vi "ACQ_Data_viewer (Module).vi"(0 "ACQ full DATA file path":path caption="File path", 5 "ChipID list":u32[](array[numeric]) format="%.0x", 7 "quants events per chip":u32[](array[numeric]), 9 "ID summary":string, 11 "ACQ events fets":u32=80 caption="Acquired events") -> ()   [LabVIEW 2015, in "VIPM2.lvlib"]
doc: "<b>Acquisition Data viewer</b>\nInclou ACQ choose Chip Data_viewer.vi"
uses:
  VIPM2.lvlib
  <vilib>/Analysis/NI_AALBase.lvlib
panel:
  out "Valid data":bool
  out "Barra Load events":i32(slide)
  in  "X scale max.":dbl=150.0 min=0.0 max=1e+29 step=10.0
  in  "X scale min.":dbl=80.0 min=0.0 max=1e+29 step=10.0
  in  "Y scale":dbl=100.0 min=5.0 max=1e+29 step=10.0
  in  "Take image button":bool
  in  "Choose Chip button":bool
  in  "Close button":bool
  out "Total number of events":u32
  out "data time":string
  out "Chip ID":string
  out "Trigger histogram 99":T1(graph)
  out "Trigger histogram 98":T1(graph)
  out "Trigger histogram 97":T1(graph)
  out "Trigger histogram 96":T1(graph)
  out "Trigger histogram 95":T1(graph)
  out "Trigger histogram 94":T1(graph)
  out "Trigger histogram 93":T1(graph)
  out "Trigger histogram 92":T1(graph)
  out "Trigger histogram 91":T1(graph)
  out "Trigger histogram 90":T1(graph)
  out "Trigger histogram 89":T1(graph)
  out "Trigger histogram 88":T1(graph)
  out "Trigger histogram 87":T1(graph)
  out "Trigger histogram 86":T1(graph)
  out "Trigger histogram 85":T1(graph)
  out "Trigger histogram 84":T1(graph)
  out "Trigger histogram 83":T1(graph)
  out "Trigger histogram 82":T1(graph)
  out "Trigger histogram 81":T1(graph)
  out "Trigger histogram 80":T1(graph)
  out "Trigger histogram 79":T1(graph)
  out "Trigger histogram 78":T1(graph)
  out "Trigger histogram 77":T1(graph)
  out "Trigger histogram 76":T1(graph)
  out "Trigger histogram 75":T1(graph)
  out "Trigger histogram 74":T1(graph)
  out "Trigger histogram 73":T1(graph)
  out "Trigger histogram 72":T1(graph)
  out "Trigger histogram 71":T1(graph)
  out "Trigger histogram 70":T1(graph)
  out "Trigger histogram 69":T1(graph)
  out "Trigger histogram 68":T1(graph)
  out "Trigger histogram 67":T1(graph)
  out "Trigger histogram 66":T1(graph)
  out "Trigger histogram 65":T1(graph)
  out "Trigger histogram 64":T1(graph)
  out "Trigger histogram 63":T1(graph)
  out "Trigger histogram 62":T1(graph)
  out "Trigger histogram 61":T1(graph)
  out "Trigger histogram 60":T1(graph)
  out "Trigger histogram 59":T1(graph)
  out "Trigger histogram 58":T1(graph)
  out "Trigger histogram 57":T1(graph)
  out "Trigger histogram 56":T1(graph)
  out "Trigger histogram 55":T1(graph)
  out "Trigger histogram 54":T1(graph)
  out "Trigger histogram 53":T1(graph)
  out "Trigger histogram 52":T1(graph)
  out "Trigger histogram 51":T1(graph)
  out "Trigger histogram 50":T1(graph)
  out "Trigger histogram 49":T1(graph)
  out "Trigger histogram 48":T1(graph)
  out "Trigger histogram 47":T1(graph)
  out "Trigger histogram 46":T1(graph)
  out "Trigger histogram 45":T1(graph)
  out "Trigger histogram 44":T1(graph)
  out "Trigger histogram 43":T1(graph)
  out "Trigger histogram 42":T1(graph)
  out "Trigger histogram 41":T1(graph)
  out "Trigger histogram 40":T1(graph)
  out "Trigger histogram 39":T1(graph)
  out "Trigger histogram 38":T1(graph)
  out "Trigger histogram 37":T1(graph)
  out "Trigger histogram 36":T1(graph)
  out "Trigger histogram 35":T1(graph)
  out "Trigger histogram 34":T1(graph)
  out "Trigger histogram 33":T1(graph)
  out "Trigger histogram 32":T1(graph)
  out "Trigger histogram 31":T1(graph)
  out "Trigger histogram 30":T1(graph)
  out "Trigger histogram 29":T1(graph)
  out "Trigger histogram 28":T1(graph)
  out "Trigger histogram 27":T1(graph)
  out "Trigger histogram 26":T1(graph)
  out "Trigger histogram 25":T1(graph)
  out "Trigger histogram 24":T1(graph)
  out "Trigger histogram 23":T1(graph)
  out "Trigger histogram 22":T1(graph)
  out "Trigger histogram 21":T1(graph)
  out "Trigger histogram 20":T1(graph)
  out "Trigger histogram 19":T1(graph)
  out "Trigger histogram 18":T1(graph)
  out "Trigger histogram 17":T1(graph)
  out "Trigger histogram 16":T1(graph)
  out "Trigger histogram 15":T1(graph)
  out "Trigger histogram 14":T1(graph)
  out "Trigger histogram 13":T1(graph)
  out "Trigger histogram 12":T1(graph)
  out "Trigger histogram 11":T1(graph)
  out "Trigger histogram 10":T1(graph)
  out "Trigger histogram 09":T1(graph)
  out "Trigger histogram 08":T1(graph)
  out "Trigger histogram 07":T1(graph)
  out "Trigger histogram 06":T1(graph)
  out "Trigger histogram 05":T1(graph)
  out "Trigger histogram 04":T1(graph)
  out "Trigger histogram 03":T1(graph)
  out "Trigger histogram 01":T1(graph)
  out "Trigger histogram 00":T1(graph)
  out "Trigger histogram 02":T1(graph)
  out "100px Trigger Data":cluster{"1px Trigger Data":u16[]}[](array[cluster])
  # "99"
  # "98"
  # "97"
  # "96"
  # "95"
  # "94"
  # "93"
  # "92"
  # "91"
  # "90"
  # "89"
  # "88"
  # "87"
  # "86"
  # "85"
  # "84"
  # "83"
  # "82"
  # "81"
  # "80"
  # "79"
  # "78"
  # "77"
  # "76"
  # "75"
  # "74"
  # "73"
  # "72"
  # "71"
  # "70"
  # "69"
  # "68"
  # "67"
  # "66"
  # "65"
  # "64"
  # "63"
  # "62"
  # "61"
  # "60"
  # "59"
  # "58"
  # "57"
  # "56"
  # "55"
  # "54"
  # "53"
  # "52"
  # "51"
  # "50"
  # "49"
  # "48"
  # "47"
  # "46"
  # "45"
  # "44"
  # "43"
  # "42"
  # "41"
  # "40"
  # "39"
  # "38"
  # "37"
  # "36"
  # "35"
  # "34"
  # "33"
  # "32"
  # "31"
  # "30"
  # "29"
  # "28"
  # "27"
  # "26"
  # "25"
  # "24"
  # "23"
  # "22"
  # "21"
  # "20"
  # "19"
  # "18"
  # "17"
  # "16"
  # "15"
  # "14"
  # "13"
  # "12"
  # "11"
  # "10"
  # "09"
  # "08"
  # "07"
  # "06"
  # "05"
  # "04"
  # "03"
  # "01"
  # "00"
  # "02"
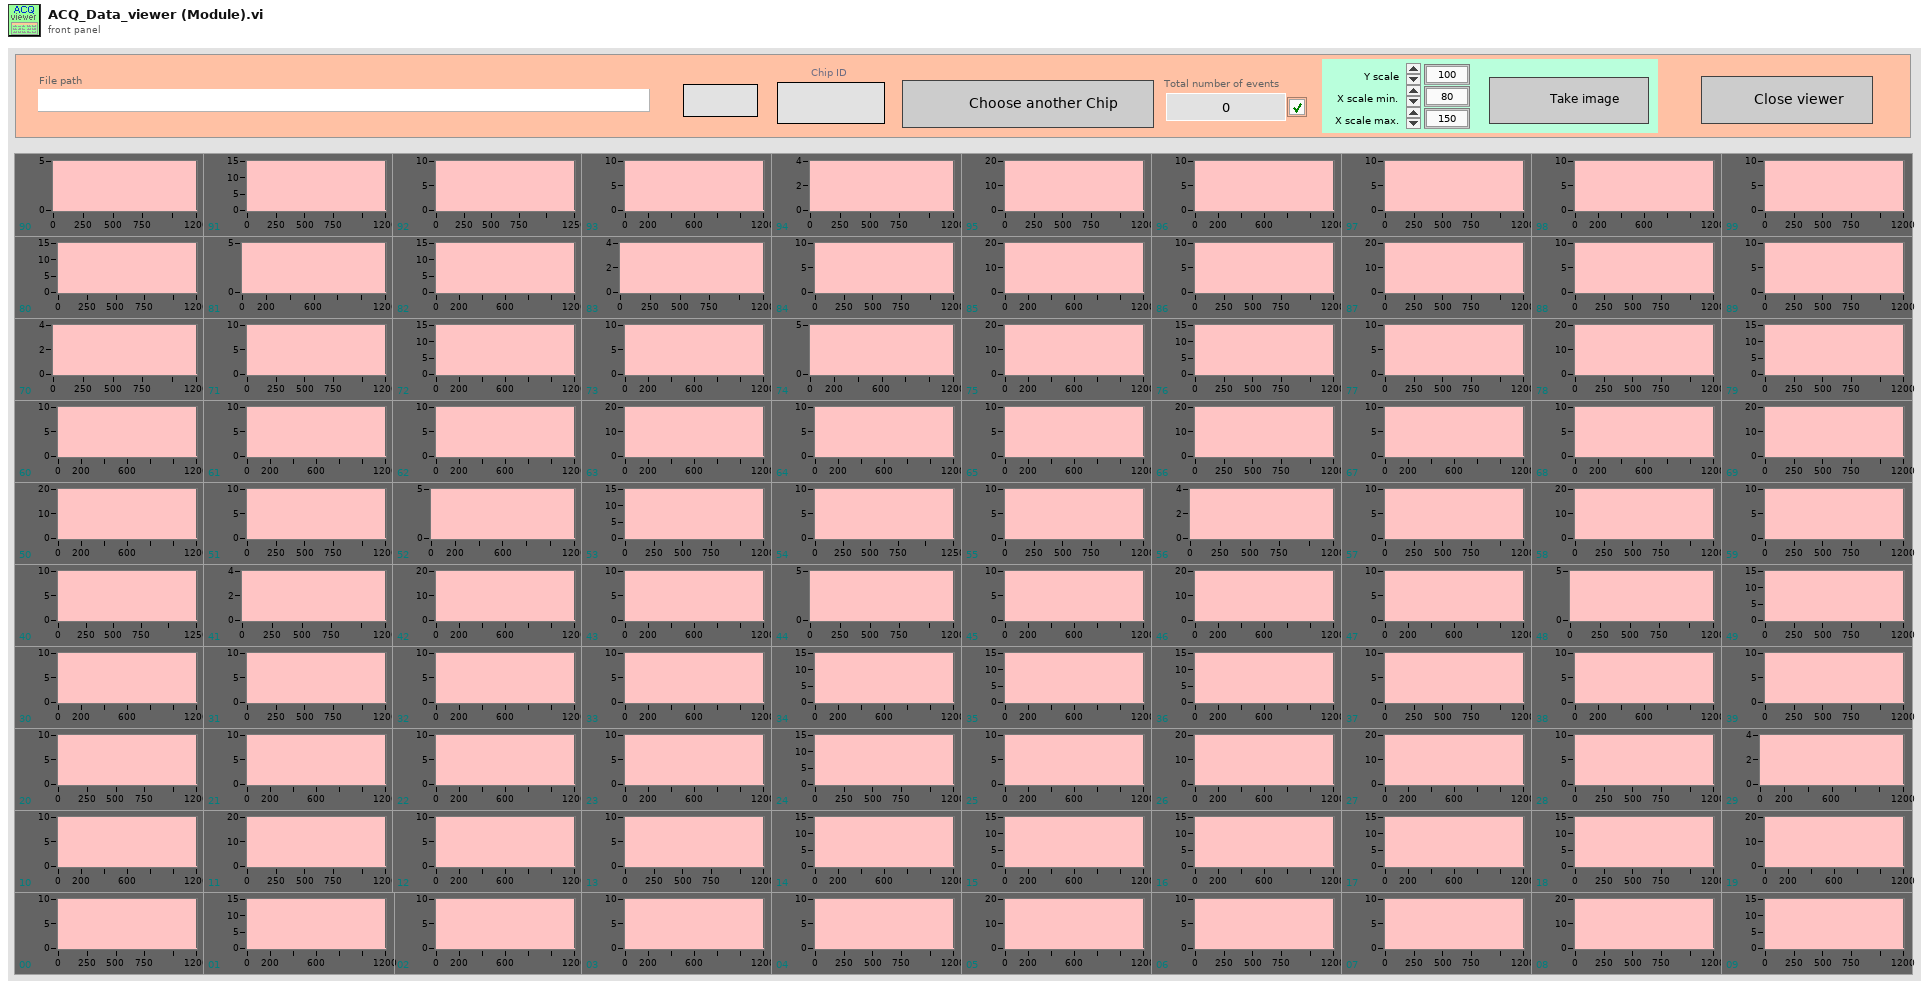
[diagram p1: front panel]
types:
  T1 = cluster{"X Values":dbl[], "Histogram: h(x)":i32[]}
  T2 = enum16{"big-endian, network order", "native, host order", "little-endian"}
  T3 = typedef "imagedata.ctl" = cluster{"image type":i32, "image depth":i32, "image":u8[], "mask":u8[], "colors":u32[], "Rectangle":cluster{"left":i16, "top":i16, "right":i16, "bottom":i16}}
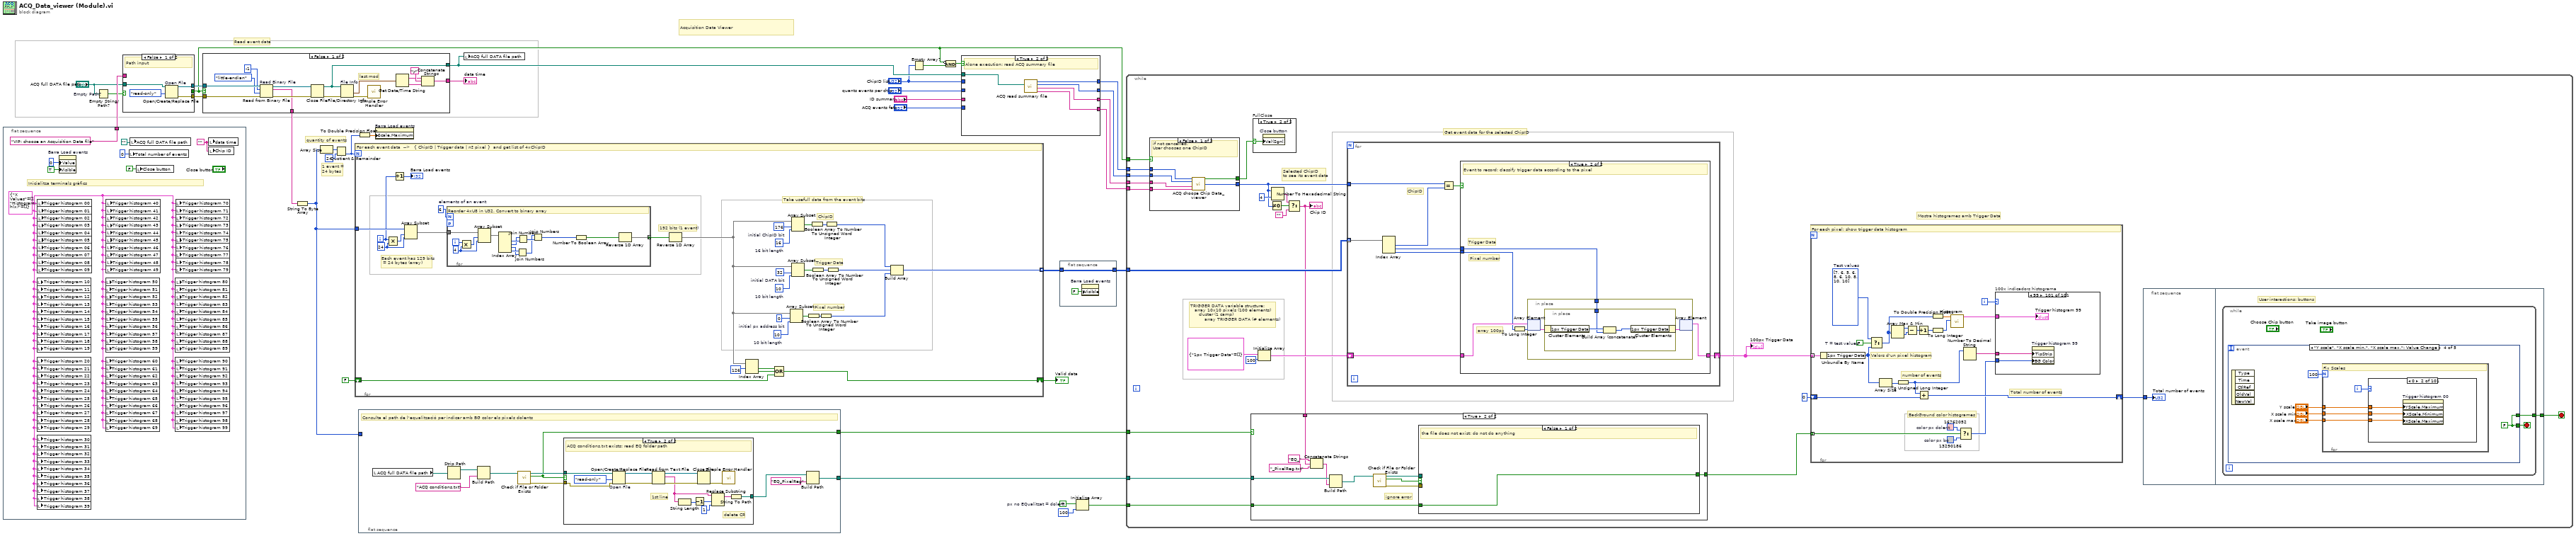
[diagram p0: block diagram]
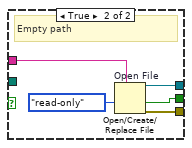
[diagram p3: hidden frame]
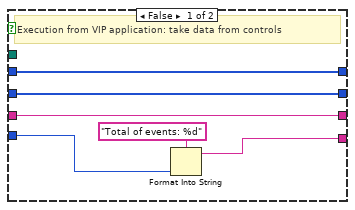
[diagram p5: hidden frame]
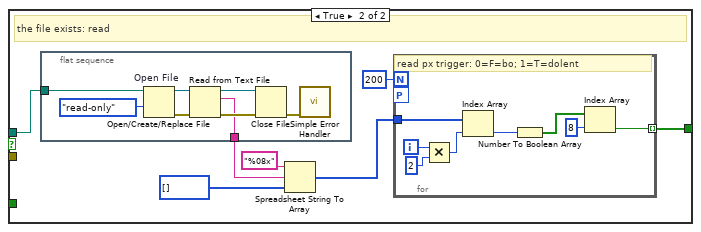
[diagram p8: hidden frame]
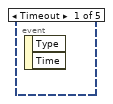
[diagram p10: hidden frame]
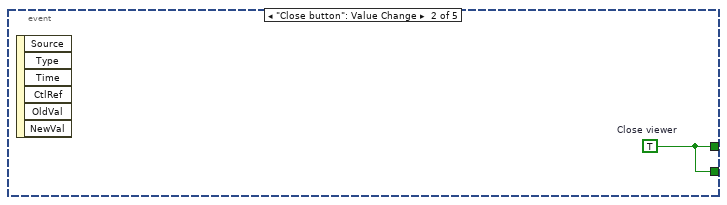
[diagram p11: hidden frame]
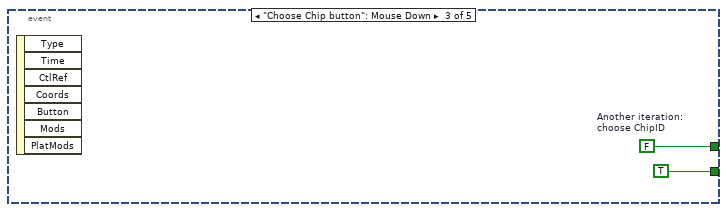
[diagram p12: hidden frame]
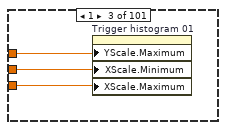
[diagram p14: hidden frame]
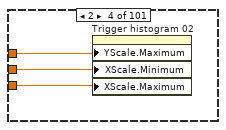
[diagram p15: hidden frame]
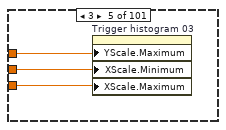
[diagram p16: hidden frame]
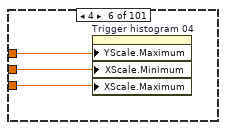
[diagram p17: hidden frame]
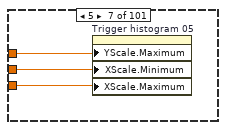
[diagram p18: hidden frame]
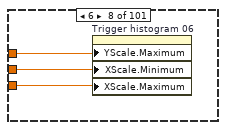
[diagram p19: hidden frame]
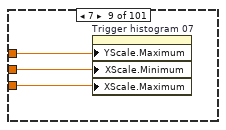
[diagram p20: hidden frame]
diagram:
  w4 = TRUE  # px no EQualitzat = dolent
  # "1 event =\n24 bytes"
  # "quantity of events"
  # "Read event data"
  # "Acquisition Data Viewer"
  n1 = flat-sequence {
    tunnel: ["VIP: choose an Acquisition Data file" ("prompt")] -> w30
    frame #0 {
      w37 = T1 {"X Values"=[], "Histogram: h(x)"=[]} ("Trigger histogram 00")
      w39 = ""
      # "Inicialitza terminals gràfics"
      n2 = local write "Trigger histogram 10"(w37) -> ()
      n3 = local write "Trigger histogram 11"(w37) -> ()
      n4 = local write "Trigger histogram 12"(w37) -> ()
      n5 = local write "Trigger histogram 13"(w37) -> ()
      n6 = local write "Trigger histogram 14"(w37) -> ()
      n7 = local write "Trigger histogram 15"(w37) -> ()
      n8 = local write "Trigger histogram 16"(w37) -> ()
      n9 = local write "Trigger histogram 17"(w37) -> ()
      n10 = local write "Trigger histogram 18"(w37) -> ()
      n11 = local write "Trigger histogram 19"(w37) -> ()
      n12 = local write "Trigger histogram 20"(w37) -> ()
      n13 = local write "Trigger histogram 21"(w37) -> ()
      n14 = local write "Trigger histogram 22"(w37) -> ()
      n15 = local write "Trigger histogram 23"(w37) -> ()
      n16 = local write "Trigger histogram 24"(w37) -> ()
      n17 = local write "Trigger histogram 25"(w37) -> ()
      n18 = local write "Trigger histogram 26"(w37) -> ()
      n19 = local write "Trigger histogram 27"(w37) -> ()
      n20 = local write "Trigger histogram 28"(w37) -> ()
      n21 = local write "Trigger histogram 29"(w37) -> ()
      n22 = local write "Trigger histogram 30"(w37) -> ()
      n23 = local write "Trigger histogram 31"(w37) -> ()
      n24 = local write "Trigger histogram 32"(w37) -> ()
      n25 = local write "Trigger histogram 33"(w37) -> ()
      n26 = local write "Trigger histogram 34"(w37) -> ()
      n27 = local write "Trigger histogram 35"(w37) -> ()
      n28 = local write "Trigger histogram 36"(w37) -> ()
      n29 = local write "Trigger histogram 37"(w37) -> ()
      n30 = local write "Trigger histogram 38"(w37) -> ()
      n31 = local write "Trigger histogram 39"(w37) -> ()
      n32 = local write "Trigger histogram 00"(w37) -> ()
      n33 = local write "Trigger histogram 01"(w37) -> ()
      n34 = local write "Trigger histogram 02"(w37) -> ()
      n35 = local write "Trigger histogram 03"(w37) -> ()
      n36 = local write "Trigger histogram 04"(w37) -> ()
      n37 = local write "Trigger histogram 05"(w37) -> ()
      n38 = local write "Trigger histogram 06"(w37) -> ()
      n39 = local write "Trigger histogram 07"(w37) -> ()
      n40 = local write "Trigger histogram 08"(w37) -> ()
      n41 = local write "Trigger histogram 09"(w37) -> ()
      n42 = property on="Barra Load events" class="Slide (strict)"("Value"=0 ("Barra Load events"), "Visible"=TRUE) -> ()  [unwired: 2 in, 2 out]
      n43 = local write "Trigger histogram 50"(w37) -> ()
      n44 = local write "Trigger histogram 51"(w37) -> ()
      n45 = local write "Trigger histogram 52"(w37) -> ()
      n46 = local write "Trigger histogram 53"(w37) -> ()
      n47 = local write "Trigger histogram 54"(w37) -> ()
      n48 = local write "Trigger histogram 55"(w37) -> ()
      n49 = local write "Trigger histogram 56"(w37) -> ()
      n50 = local write "Trigger histogram 57"(w37) -> ()
      n51 = local write "Trigger histogram 58"(w37) -> ()
      n52 = local write "Trigger histogram 59"(w37) -> ()
      n53 = local write "Trigger histogram 60"(w37) -> ()
      n54 = local write "Trigger histogram 61"(w37) -> ()
      n55 = local write "Trigger histogram 62"(w37) -> ()
      n56 = local write "Trigger histogram 63"(w37) -> ()
      n57 = local write "Trigger histogram 64"(w37) -> ()
      n58 = local write "Trigger histogram 65"(w37) -> ()
      n59 = local write "Trigger histogram 66"(w37) -> ()
      n60 = local write "Trigger histogram 67"(w37) -> ()
      n61 = local write "Trigger histogram 68"(w37) -> ()
      n62 = local write "Trigger histogram 69"(w37) -> ()
      n63 = local write "Trigger histogram 40"(w37) -> ()
      n64 = local write "Trigger histogram 41"(w37) -> ()
      n65 = local write "Trigger histogram 42"(w37) -> ()
      n66 = local write "Trigger histogram 43"(w37) -> ()
      n67 = local write "Trigger histogram 44"(w37) -> ()
      n68 = local write "Trigger histogram 45"(w37) -> ()
      n69 = local write "Trigger histogram 46"(w37) -> ()
      n70 = local write "Trigger histogram 47"(w37) -> ()
      n71 = local write "Trigger histogram 48"(w37) -> ()
      n72 = local write "Trigger histogram 49"(w37) -> ()
      n73 = local write "Total number of events"(u32 0 ("Total number of events")) -> ()
      n74 = local write "ACQ full DATA file path"(path "") -> ()
      n75 = local write "Close button"(FALSE ("Close button")) -> ()
      n76 = local write "Trigger histogram 80"(w37) -> ()
      n77 = local write "Trigger histogram 81"(w37) -> ()
      n78 = local write "Trigger histogram 82"(w37) -> ()
      n79 = local write "Trigger histogram 83"(w37) -> ()
      n80 = local write "Trigger histogram 84"(w37) -> ()
      n81 = local write "Trigger histogram 85"(w37) -> ()
      n82 = local write "Trigger histogram 86"(w37) -> ()
      n83 = local write "Trigger histogram 87"(w37) -> ()
      n84 = local write "Trigger histogram 88"(w37) -> ()
      n85 = local write "Trigger histogram 89"(w37) -> ()
      n86 = local write "Trigger histogram 90"(w37) -> ()
      n87 = local write "Trigger histogram 91"(w37) -> ()
      n88 = local write "Trigger histogram 92"(w37) -> ()
      n89 = local write "Trigger histogram 93"(w37) -> ()
      n90 = local write "Trigger histogram 94"(w37) -> ()
      n91 = local write "Trigger histogram 95"(w37) -> ()
      n92 = local write "Trigger histogram 96"(w37) -> ()
      n93 = local write "Trigger histogram 97"(w37) -> ()
      n94 = local write "Trigger histogram 98"(w37) -> ()
      n95 = local write "Trigger histogram 99"(w37) -> ()
      n96 = local write "Trigger histogram 70"(w37) -> ()
      n97 = local write "Trigger histogram 71"(w37) -> ()
      n98 = local write "Trigger histogram 72"(w37) -> ()
      n99 = local write "Trigger histogram 73"(w37) -> ()
      n100 = local write "Trigger histogram 74"(w37) -> ()
      n101 = local write "Trigger histogram 75"(w37) -> ()
      n102 = local write "Trigger histogram 76"(w37) -> ()
      n103 = local write "Trigger histogram 77"(w37) -> ()
      n104 = local write "Trigger histogram 78"(w37) -> ()
      n105 = local write "Trigger histogram 79"(w37) -> ()
      n106 = local write "data time"(w39) -> ()
      n107 = local write "Chip ID"(w39) -> ()
    }
  }
  n108 = Empty String/Path? "Empty Path?"(string/path="ACQ full DATA file path") -> (empty?=w29:bool)
  n109 = case shown="False" w29 {
    tunnel: [w44 w49] -> w33
    tunnel: [w43 w48] -> w32
    tunnel: [_ w47] -> w9
    tunnel: w30 -> [_ w46]
    tunnel: "ACQ full DATA file path" -> [w42 _]
    frame False {
      # "Path input"
      n110 = Open/Create/Replace File "Open File"(file path (use dialog)=w42, access (0:read/write)=enum16{"read/write", "read-only", "write-only"}."read-only") -> (refnum out=w43:refnum<file>, error out=w44:errorcluster)  [unwired: 4 in, 1 out]
    }
    frame True {
      # "Empty path"
      n111 = Open/Create/Replace File "Open File"(prompt=w46, access (0:read/write)=enum16{"read/write", "read-only", "write-only"}."read-only") -> (refnum out=w48:refnum<file>, cancelled=w47:bool, error out=w49:errorcluster)  [unwired: 4 in]
    }
  }
  n112 = case shown="False" w9 {
    tunnel: w33 -> [w65 _]
    tunnel: w32 -> [w64 _]
    tunnel: [w59 _] -> w25
    tunnel: [w52 _] -> w31
    tunnel: [w51 _] -> w20
    frame False {
      # "last mod"
      n113 = Read from Binary File "Read Binary File"(8:w65, 9:T2."little-endian" ("byte order (0:big-endian, network order)"), 10:-1 ("count (1)"), 11:w64) -> (0:w62:errorcluster, 2:w59:string, 3:w61:refnum<file>)  [unwired: 2 in, 1 out]
      n114 = Close File(refnum=w61, error in=w62) -> (path=w51:path, error out=w58:errorcluster)
      n115 = File/Directory Info "File Info"(path=w51, error in=w58) -> (last mod=w53:timestamp, error out=w57:errorcluster)  [unwired: 5 out]
      n116 = call <vilib>:"Simple Error Handler.vi"("error in (no error)"=w57) -> ()  [unwired: 4 in, 5 out]
      n117 = Get Date/Time String(seconds (now)=w53) -> (date string=w54:string, time string=w56:string)  [unwired: 2 in]
      n118 = Concatenate Strings(w54, "\r", w56) -> (w52:string)
    }
    frame True {
      # "Openning cancelled"
    }
  }
  "data time" <- w31
  n119 = String To Byte Array(string=w25) -> (unsigned byte array=w8:u8[])
  n120 = Array Size(array=w8) -> (size(s)=w26:i32)
  n121 = Quotient & Remainder(x=w26, y=24) -> (floor(x/y)=w23:i32)  [unwired: 1 out]
  n122 = for {
    N: w23 -> [_]
    tunnel: w8 -> [w91]
    tunnel: [w74] -> w21 mode=indexing
    shift-right: [w66] -> w1
    shift-left: FALSE -> [w67]
    i -> [w72]
    w80 = 10  # 10 bit length
    w81 = 0  # initial px address bit
    w85 = 10  # 10 bit length
    w84 = 32  # initial DATA bit
    w88 = 16  # 16 bit length
    w89 = 176  # initial ChipID bit
    w94 = 24 ("y")
    w95 = 6  # elements of an event
    # "Take usefull data from the event bits"
    # "Pixel number"
    # "Trigger Data"
    # "ChipID"
    # "192 bits (1 event)"
    # "Each event has 129 bits\n = 24 bytes (array)"
    # "For each event data  -->   { ChipID | Trigger data | nº pixel }  and get list of 4xChipID"
    n123 = Multiply(x=w72, y=w94) -> (x*y=w93:i32)
    n124 = Increment(x=w72) -> (x+1=→"Barra Load events":i32)
    n125 = Array Subset "Array Subset"(array=w91, index=w93, length=w94) -> (w92:u8[])
    n126 = for {
      N: w95 -> [_]
      tunnel: w92 -> [w108]
      workers-P: _ -> [_]
      tunnel: [w96] -> w90 mode=concatenating
      i -> [w109]
      w106 = 4 ("y")
      # "Reorder 4xU8 in U32. Convert to binary array"
      n127 = Multiply(x=w109, y=w106) -> (x*y=w107:i32)
      n128 = Array Subset "Array Subset"(array=w108, index=w107, length=w106) -> (w105:u8[])
      n129 = Index Array(array=w105) -> (element #1=w104:u8, element #2=w103:u8, element #3=w101:u8, element #4=w102:u8)  [unwired: 4 in]
      n130 = Join Numbers(hi=w102, lo=w101) -> ((hi.lo)=w99:u16)
      n131 = Join Numbers(hi=w103, lo=w104) -> ((hi.lo)=w100:u16)
      n132 = Join Numbers(hi=w99, lo=w100) -> ((hi.lo)=w97:u32)
      n133 = Number To Boolean Array(number=w97) -> (Boolean array=w98:bool[])
      n134 = Reverse 1D Array(array=w98) -> (reversed array=w96:bool[])
    }
    n135 = Reverse 1D Array(array=w90) -> (reversed array=w71:bool[])
    n136 = Index Array(array=w71, index #1=126 ("index")) -> (element #1=w69:bool, element #2=w68:bool)  [unwired: 1 in]
    n137 = Compound Arithmetic op=OR(w69, w68, w67) -> (w66:bool)
    n138 = Array Subset "Array Subset"(array=w71, index=w81, length=w80) -> (w79:bool[])
    n139 = Array Subset "Array Subset"(array=w71, index=w89, length=w88) -> (w87:bool[])
    n140 = Array Subset "Array Subset"(array=w71, index=w84, length=w85) -> (w82:bool[])
    n141 = Boolean Array To Number(Boolean array=w79) -> (number=w78:u32)
    n142 = Boolean Array To Number(Boolean array=w87) -> (number=w86:u32)
    n143 = Boolean Array To Number(Boolean array=w82) -> (number=w83:u32)
    n144 = To Unsigned Word Integer(number=w78) -> (unsigned 16bit integer=w75:u16)
    n145 = To Unsigned Word Integer(number=w86) -> (unsigned 16bit integer=w77:u16)
    n146 = To Unsigned Word Integer(number=w83) -> (unsigned 16bit integer=w76:u16)
    n147 = Build Array "Build Array"(w77, w76, w75) -> (w74:u16[])
  }
  "Valid data" <- w1
  n148 = To Double Precision Float(number=w23) -> (double precision float=w24:dbl)
  n149 = flat-sequence {
    tunnel: w8 -> [_]
    tunnel: [w110] -> w7
    tunnel: [w113] -> w6
    frame #0 {
      # "Consulta el path de l'equalització per indicar amb BG color els pixels dolents"
      n150 = local read "ACQ full DATA file path"() -> (w114:path)
      n151 = Strip Path(path=w114) -> (stripped path=w115:path)  [unwired: 1 out]
      n152 = Build Path(base path=w115, name or relative path="ACQ conditions.txt") -> (appended path=w117:path)
      n153 = call <vilib>:"Check if File or Folder Exists.vi"("path"=w117) -> ("error out"=w119:errorcluster, "file or folder exists?"=w113:bool, "dup path"=w118:path)  [unwired: 8 in]
      n154 = case shown="True" w113 {
        tunnel: w118 -> [_ w133]
        tunnel: w119 -> [_ w131]
        tunnel: [_ w125] -> w112
        frame False {
          # "ACQ conditions.txt doesn't exist"
        }
        frame True {
          # "delete CR"
          # "1st line"
          # "ACQ conditions.txt exists: read EQ folder path"
          n155 = Open/Create/Replace File "Open File"(file path (use dialog)=w133, error in=w131, access (0:read/write)=enum16{"read/write", "read-only", "write-only"}."read-only") -> (refnum out=w130:refnum<file>, error out=w129:errorcluster)  [unwired: 3 in, 1 out]
          n156 = Read from Text File(file (use dialog)=w130, error in=w129) -> (refnum out=w128:refnum<file>, text=w124:string, error out=w127:errorcluster)  [unwired: 2 in, 1 out]
          n157 = String Length(string=w124) -> (length=w123:i32)
          n158 = Decrement(x=w123) -> (x-1=w122:i32)
          n159 = Close File(refnum=w128, error in=w127) -> (error out=w126:errorcluster)  [unwired: 1 out]
          n160 = Replace Substring(2:1 ("length (len. of substring)"), 3:w122, 5:w124) -> (1:w120:string)  [unwired: 1 in, 1 out]
          n161 = call <vilib>:"Simple Error Handler.vi"("error in (no error)"=w126) -> ()  [unwired: 4 in, 5 out]
          n162 = String To Path(string=w120) -> (path=w125:path)
        }
      }
      n163 = Build Path(base path=w112, name or relative path="EQ_PixelReg") -> (appended path=w110:path)
    }
  }
  n164 = property on="Barra Load events" class="Slide (strict)"("Scale.Maximum"=w24) -> ()  [unwired: 2 in, 2 out]
  n165 = local write "ACQ full DATA file path"(w20) -> ()
  n166 = Empty Array?(array="ChipID list") -> (empty?=w11:bool)
  n167 = Compound Arithmetic op=AND(invert w9, w11) -> (w10:bool)
  n168 = case shown="True" w10 {
    tunnel: w20 -> [_ w144]
    tunnel: "ChipID list" -> [w139 _]
    tunnel: [w139 w143] -> w12
    tunnel: [w138 w142] -> w13
    tunnel: "quants events per chip" -> [w138 _]
    tunnel: "ID summary" -> [w137 _]
    tunnel: "ACQ events fets" -> [w135 _]
    tunnel: [w137 w141] -> w14
    tunnel: [w134 w140] -> w15
    frame False {
      # "Execution from VIP application: take data from controls"
      n169 = Format Into String "Format Into String"(format string="Total of events: %d", w135) -> (resulting string=w134:string)  [unwired: 2 in, 1 out]
    }
    frame True {
      # "Alone execution: read ACQ summary file"
      n170 = call "ACQ read summary file.vi"("ACQ binary data file path"=w144) -> ("Total of events"=w140:string, "ID summary"=w141:string, "quants events per chip"=w142:u32[], "ChipID list"=w143:u32[])  [unwired: 7 in]
    }
  }
  n171 = flat-sequence {
    tunnel: [w146] -> w22
    tunnel: w21 -> [w146]
    frame #0 {
      n172 = property on="Barra Load events" class="Slide (strict)"("Visible"=FALSE) -> ()  [unwired: 2 in, 2 out]
    }
  }
  n173 = Initialize Array "Initialize Array"(w4, 100 ("dimension size")) -> (w3:bool[])
  n174 = while {
    tunnel: w22 -> [w170]
    tunnel: w15 -> [w157]
    tunnel: w14 -> [w156]
    tunnel: w13 -> [w155]
    tunnel: w12 -> [w154]
    tunnel: w9 -> [w153]
    tunnel: w7 -> [w152]
    tunnel: w6 -> [w149]
    tunnel: w3 -> [w148]
    stop <- w164 stop-if-true
    # "Mostra histogrames amb Trigger Data"
    # "TRIGGER DATA variable structure:\n   array 10x10 pixels (100 elements)\n      cluster (1 camp)\n          array TRIGGER DATA (# elements)"
    # "Get event data for the selected ChipID"
    # "Selected ChipID\nto see its event data"
    n175 = case shown="False" w153 {
      selector: w153 -> [_ w214]
      tunnel: [w213 _] -> w158
      tunnel: w157 -> [w212 _]
      tunnel: w156 -> [w211 _]
      tunnel: w155 -> [w210 _]
      tunnel: w154 -> [w209 _]
      tunnel: [w208 w214] -> w147
      frame False {
        # "if not cancelled,\nUser chooses one ChipID"
        n176 = call "ACQ choose Chip Data_viewer.vi"("Chip ID list"=w209, "quants events per Chip"=w210, "summary IDs"=w211, "Total of events"=w212) -> ("FullClose"=w208:bool, "ChipID choosed"=w213:u16)  [unwired: 10 in]
      }
      frame True {
      }
    }
    n177 = case "FullClose" shown="True" w147 {
      selector: w147 -> [_ w171]
      frame False {
      }
      frame True {
        n178 = property on="Close button" class="Bool (strict)"("Val(Sgnl)"=w171) -> ()  [unwired: 2 in, 2 out]
      }
    }
    n179 = Initialize Array "Initialize Array"(cluster{"1px Trigger Data":u16[]} {"1px Trigger Data"=[]} ("1px Trigger Data"), 100 ("dimension size")) -> (w167:cluster{"1px Trigger Data":u16[]}[])
    n180 = Not Equal To 0?(x=w158) -> (x != 0?=w161:bool)
    n181 = Number To Hexadecimal String(1:i16 4 ("width (-)"), 2:w158) -> (0:w162:string)
    n182 = Select(t=w162, s=w161, f="") -> (s? t:f=w151:string)
    "Chip ID" <- w151
    n183 = case shown="True" w149 {
      tunnel: w152 -> [_ w183]
      tunnel: w151 -> [_ w181]
      tunnel: [w172 w174] -> w150
      tunnel: w148 -> [w172 w173]
      frame False {
      }
      frame True {
        # "ignore error"
        n184 = Concatenate Strings "Concatenate Strings"("EQ_", w181, "_PixelReg.txt") -> (w179:string)
        n185 = Build Path(base path=w183, name or relative path=w179) -> (appended path=w178:path)
        n186 = call <vilib>:"Check if File or Folder Exists.vi"("path"=w178) -> ("error out"=w175:errorcluster, "file or folder exists?"=w176:bool, "dup path"=w177:path)  [unwired: 8 in]
        n187 = case shown="False" w176 {
          tunnel: w177 -> [_ w191]
          tunnel: w175 -> [_ _]
          tunnel: [w184 w185] -> w174
          tunnel: w173 -> [w184 _]
          frame False {
            # "the file does not exist: do not do anything"
          }
          frame True {
            # "the file exists: read"
            n188 = flat-sequence {
              tunnel: w191 -> [w207]
              tunnel: [w200] -> w190
              frame #0 {
                n189 = Open/Create/Replace File "Open File"(file path (use dialog)=w207, access (0:read/write)=enum16{"read/write", "read-only", "write-only"}."read-only") -> (refnum out=w204:refnum<file>, error out=w205:errorcluster)  [unwired: 4 in, 1 out]
                n190 = Read from Text File(file (use dialog)=w204, error in=w205) -> (refnum out=w203:refnum<file>, text=w200:string, error out=w202:errorcluster)  [unwired: 2 in, 1 out]
                n191 = Close File(refnum=w203, error in=w202) -> (error out=w201:errorcluster)  [unwired: 1 out]
                n192 = call <vilib>:"Simple Error Handler.vi"("error in (no error)"=w201) -> ()  [unwired: 4 in, 5 out]
              }
            }
            n193 = Spreadsheet String To Array(format string="%08x", spreadsheet string=w190, array type (2D Dbl)=u32[] []) -> (array=w187:u32[])  [unwired: 1 in]
            n194 = for {
              N: 200 -> [_]
              tunnel: w187 -> [w196]
              tunnel: [w192] -> w185 mode=indexing
              workers-P: _ -> [_]
              i -> [w199]
              # "read px trigger: 0=F=bo; 1=T=dolent"
              n195 = Multiply(x=w199, y=2) -> (x*y=w197:i32)
              n196 = Index Array "Index Array"(array=w196, index=w197) -> (element=w195:u32)
              n197 = Number To Boolean Array(number=w195) -> (Boolean array=w194:bool[])
              n198 = Index Array "Index Array"(array=w194, index=8) -> (element=w192:bool)
            }
          }
        }
      }
    }
    n199 = for {
      tunnel: w170 -> [w870] mode=indexing
      tunnel: w158 -> [w874]
      shift-right: [w871] -> w159
      shift-left: w167 -> [w872]
      # "ChipID"
      n200 = Index Array "Index Array"(array=w870) -> (element #1=w867:u16, element #2=w869:u16, element #3=w868:u16)  [unwired: 3 in]
      n201 = Equal?(x=w874, y=w867) -> (x = y?=w873:bool)
      n202 = case shown="True" w873 {
        tunnel: w872 -> [w875 w880]
        tunnel: [w875 w879] -> w871
        tunnel: w869 -> [_ w878]
        tunnel: w868 -> [_ w876]
        frame False {
          # "This event is not from selected ChipID: skip"
        }
        frame True {
          # "array 100px"
          # "Pixel number"
          # "Trigger Data"
          # "Event to record: classify trigger data according to the pixel"
          n203 = To Long Integer(number=w876) -> (32bit integer=w877:i32)
          n204 = in-place {
            in-place-border: w878 -> [w881]
            n205 = in-place-array #1(w880, w877) -> (w883:cluster{"1px Trigger Data":u16[]})
            n206 = in-place {
              in-place-border: w881 -> [w885]
              n207 = in-place-cluster #2(w883) -> ("1px Trigger Data"=w886:u16[])
              n208 = Build Array (concatenate) "Build Array"(w886, w885) -> (w884:u16[])
              n209 = in-place-cluster #2("1px Trigger Data"=w884) -> (w882:cluster{"1px Trigger Data":u16[]})
            }
            n210 = in-place-array #1(w882) -> (w879:cluster{"1px Trigger Data":u16[]}[])  [unwired: 1 out]
          }
        }
      }
    }
    "100px Trigger Data" <- w159
    n211 = for {
      tunnel: w159 -> [w560] mode=indexing
      shift-right: [w553] -> w165
      shift-left: u32 0 -> [w552]
      tunnel: w150 -> [w546] mode=indexing
      i -> [w559]
      w548 = u32 13290186  # color px bo
      w547 = u32 16762052  # color px dolent
      w556 = u16[] [7, 6, 5, 6, 8, 6, 10, 8, 10, 10]  # Test values
      w555 = FALSE  # T = test values
      # "BackGround color histogrames"
      # "Total number of events"
      # "number of events"
      # "Valors d'un pixel histogram"
      # "For each pixel: show trigger data histogram"
      n212 = Unbundle By Name(w560) -> ("1px Trigger Data"=w554:u16[])
      n213 = Select(t=w556, s=w555, f=w554) -> (s? t:f=w557:u16[])
      n214 = Array Size(array=w554) -> (size(s)=w551:i32)
      n215 = Array Max & Min(array=w557) -> (max value=w563:u16, min value=w562:u16)  [unwired: 2 out]
      n216 = To Unsigned Long Integer(number=w551) -> (unsigned 32bit integer=w550:u32)
      n217 = Subtract(x=w563, y=w562) -> (x-y=w561:u16)
      n218 = Increment(x=w561) -> (x+1=w565:u16)
      n219 = Add(x=w550, y=w552) -> (x+y=w553:u32)
      n220 = To Long Integer(number=w565) -> (32bit integer=w566:i32)
      n221 = To Double Precision Float(number=w557) -> (double precision float=w564:dbl[])
      n222 = call <vilib>:"Histogram.vi"("intervals"=w566, "X"=w564) -> ("Histogram Graph"=w558:T1)  [unwired: 6 in, 3 out]
      n223 = Select(t=w547, s=w546, f=w548) -> (s? t:f=w545:u32)
      n224 = Number To Decimal String(number=w550) -> (decimal integer string=w549:string)  [unwired: 1 in]
      n225 = case "100x indicadors histograma" shown="99" w559 {
        tunnel: w558 -> [_ w569 w572 w575 w578 w581 w584 w587 w590 w593 w596 w599 w602 w605 w608 w611 w614 w617 w620 w623 w626 w629 w632 w635 w638 w641 w644 w647 w650 w653 w656 w659 w662 w665 w668 w671 w674 w677 w680 w683 w686 w689 w692 w695 w698 w701 w704 w707 w710 w713 w716 w719 w722 w725 w728 w731 w734 w737 w740 w743 w746 w749 w752 w755 w758 w761 w764 w767 w770 w773 w776 w779 w782 w785 w788 w791 w794 w797 w800 w803 w806 w809 w812 w815 w818 w821 w824 w827 w830 w833 w836 w839 w842 w845 w848 w851 w854 w857 w860 w863 w866]
        tunnel: w549 -> [_ w568 w571 w574 w577 w580 w583 w586 w589 w592 w595 w598 w601 w604 w607 w610 w613 w616 w619 w622 w625 w628 w631 w634 w637 w640 w643 w646 w649 w652 w655 w658 w661 w664 w667 w670 w673 w676 w679 w682 w685 w688 w691 w694 w697 w700 w703 w706 w709 w712 w715 w718 w721 w724 w727 w730 w733 w736 w739 w742 w745 w748 w751 w754 w757 w760 w763 w766 w769 w772 w775 w778 w781 w784 w787 w790 w793 w796 w799 w802 w805 w808 w811 w814 w817 w820 w823 w826 w829 w832 w835 w838 w841 w844 w847 w850 w853 w856 w859 w862 w865]
        tunnel: w545 -> [_ w567 w570 w573 w576 w579 w582 w585 w588 w591 w594 w597 w600 w603 w606 w609 w612 w615 w618 w621 w624 w627 w630 w633 w636 w639 w642 w645 w648 w651 w654 w657 w660 w663 w666 w669 w672 w675 w678 w681 w684 w687 w690 w693 w696 w699 w702 w705 w708 w711 w714 w717 w720 w723 w726 w729 w732 w735 w738 w741 w744 w747 w750 w753 w756 w759 w762 w765 w768 w771 w774 w777 w780 w783 w786 w789 w792 w795 w798 w801 w804 w807 w810 w813 w816 w819 w822 w825 w828 w831 w834 w837 w840 w843 w846 w849 w852 w855 w858 w861 w864]
        frame Default {
        }
        frame 0 {
          n226 = property on="Trigger histogram 00" class="XYGraph (strict)"("TipStrip"=w568, "BG Color"=w567) -> ()  [unwired: 2 in, 2 out]
          "Trigger histogram 00" <- w569
        }
        frame 1 {
          n227 = property on="Trigger histogram 01" class="XYGraph (strict)"("TipStrip"=w571, "BG Color"=w570) -> ()  [unwired: 2 in, 2 out]
          "Trigger histogram 01" <- w572
        }
        frame 2 {
          n228 = property on="Trigger histogram 02" class="XYGraph (strict)"("TipStrip"=w574, "BG Color"=w573) -> ()  [unwired: 2 in, 2 out]
          "Trigger histogram 02" <- w575
        }
        frame 3 {
          n229 = property on="Trigger histogram 03" class="XYGraph (strict)"("TipStrip"=w577, "BG Color"=w576) -> ()  [unwired: 2 in, 2 out]
          "Trigger histogram 03" <- w578
        }
        frame 4 {
          n230 = property on="Trigger histogram 04" class="XYGraph (strict)"("TipStrip"=w580, "BG Color"=w579) -> ()  [unwired: 2 in, 2 out]
          "Trigger histogram 04" <- w581
        }
        frame 5 {
          n231 = property on="Trigger histogram 05" class="XYGraph (strict)"("TipStrip"=w583, "BG Color"=w582) -> ()  [unwired: 2 in, 2 out]
          "Trigger histogram 05" <- w584
        }
        frame 6 {
          n232 = property on="Trigger histogram 06" class="XYGraph (strict)"("TipStrip"=w586, "BG Color"=w585) -> ()  [unwired: 2 in, 2 out]
          "Trigger histogram 06" <- w587
        }
        frame 7 {
          n233 = property on="Trigger histogram 07" class="XYGraph (strict)"("TipStrip"=w589, "BG Color"=w588) -> ()  [unwired: 2 in, 2 out]
          "Trigger histogram 07" <- w590
        }
        frame 8 {
          n234 = property on="Trigger histogram 08" class="XYGraph (strict)"("TipStrip"=w592, "BG Color"=w591) -> ()  [unwired: 2 in, 2 out]
          "Trigger histogram 08" <- w593
        }
        frame 9 {
          n235 = property on="Trigger histogram 09" class="XYGraph (strict)"("TipStrip"=w595, "BG Color"=w594) -> ()  [unwired: 2 in, 2 out]
          "Trigger histogram 09" <- w596
        }
        frame 10 {
          n236 = property on="Trigger histogram 10" class="XYGraph (strict)"("TipStrip"=w598, "BG Color"=w597) -> ()  [unwired: 2 in, 2 out]
          "Trigger histogram 10" <- w599
        }
        frame 11 {
          n237 = property on="Trigger histogram 11" class="XYGraph (strict)"("TipStrip"=w601, "BG Color"=w600) -> ()  [unwired: 2 in, 2 out]
          "Trigger histogram 11" <- w602
        }
        frame 12 {
          n238 = property on="Trigger histogram 12" class="XYGraph (strict)"("TipStrip"=w604, "BG Color"=w603) -> ()  [unwired: 2 in, 2 out]
          "Trigger histogram 12" <- w605
        }
        frame 13 {
          n239 = property on="Trigger histogram 13" class="XYGraph (strict)"("TipStrip"=w607, "BG Color"=w606) -> ()  [unwired: 2 in, 2 out]
          "Trigger histogram 13" <- w608
        }
        frame 14 {
          n240 = property on="Trigger histogram 14" class="XYGraph (strict)"("TipStrip"=w610, "BG Color"=w609) -> ()  [unwired: 2 in, 2 out]
          "Trigger histogram 14" <- w611
        }
        frame 15 {
          n241 = property on="Trigger histogram 15" class="XYGraph (strict)"("TipStrip"=w613, "BG Color"=w612) -> ()  [unwired: 2 in, 2 out]
          "Trigger histogram 15" <- w614
        }
        frame 16 {
          n242 = property on="Trigger histogram 16" class="XYGraph (strict)"("TipStrip"=w616, "BG Color"=w615) -> ()  [unwired: 2 in, 2 out]
          "Trigger histogram 16" <- w617
        }
        frame 17 {
          n243 = property on="Trigger histogram 17" class="XYGraph (strict)"("TipStrip"=w619, "BG Color"=w618) -> ()  [unwired: 2 in, 2 out]
          "Trigger histogram 17" <- w620
        }
        frame 18 {
          n244 = property on="Trigger histogram 18" class="XYGraph (strict)"("TipStrip"=w622, "BG Color"=w621) -> ()  [unwired: 2 in, 2 out]
          "Trigger histogram 18" <- w623
        }
        frame 19 {
          n245 = property on="Trigger histogram 19" class="XYGraph (strict)"("TipStrip"=w625, "BG Color"=w624) -> ()  [unwired: 2 in, 2 out]
          "Trigger histogram 19" <- w626
        }
        frame 20 {
          n246 = property on="Trigger histogram 20" class="XYGraph (strict)"("TipStrip"=w628, "BG Color"=w627) -> ()  [unwired: 2 in, 2 out]
          "Trigger histogram 20" <- w629
        }
        frame 21 {
          n247 = property on="Trigger histogram 21" class="XYGraph (strict)"("TipStrip"=w631, "BG Color"=w630) -> ()  [unwired: 2 in, 2 out]
          "Trigger histogram 21" <- w632
        }
        frame 22 {
          n248 = property on="Trigger histogram 22" class="XYGraph (strict)"("TipStrip"=w634, "BG Color"=w633) -> ()  [unwired: 2 in, 2 out]
          "Trigger histogram 22" <- w635
        }
        frame 23 {
          n249 = property on="Trigger histogram 23" class="XYGraph (strict)"("TipStrip"=w637, "BG Color"=w636) -> ()  [unwired: 2 in, 2 out]
          "Trigger histogram 23" <- w638
        }
        frame 24 {
          n250 = property on="Trigger histogram 24" class="XYGraph (strict)"("TipStrip"=w640, "BG Color"=w639) -> ()  [unwired: 2 in, 2 out]
          "Trigger histogram 24" <- w641
        }
        frame 25 {
          n251 = property on="Trigger histogram 25" class="XYGraph (strict)"("TipStrip"=w643, "BG Color"=w642) -> ()  [unwired: 2 in, 2 out]
          "Trigger histogram 25" <- w644
        }
        frame 26 {
          n252 = property on="Trigger histogram 26" class="XYGraph (strict)"("TipStrip"=w646, "BG Color"=w645) -> ()  [unwired: 2 in, 2 out]
          "Trigger histogram 26" <- w647
        }
        frame 27 {
          n253 = property on="Trigger histogram 27" class="XYGraph (strict)"("TipStrip"=w649, "BG Color"=w648) -> ()  [unwired: 2 in, 2 out]
          "Trigger histogram 27" <- w650
        }
        frame 28 {
          n254 = property on="Trigger histogram 28" class="XYGraph (strict)"("TipStrip"=w652, "BG Color"=w651) -> ()  [unwired: 2 in, 2 out]
          "Trigger histogram 28" <- w653
        }
        frame 29 {
          n255 = property on="Trigger histogram 29" class="XYGraph (strict)"("TipStrip"=w655, "BG Color"=w654) -> ()  [unwired: 2 in, 2 out]
          "Trigger histogram 29" <- w656
        }
        frame 30 {
          n256 = property on="Trigger histogram 30" class="XYGraph (strict)"("TipStrip"=w658, "BG Color"=w657) -> ()  [unwired: 2 in, 2 out]
          "Trigger histogram 30" <- w659
        }
        frame 31 {
          n257 = property on="Trigger histogram 31" class="XYGraph (strict)"("TipStrip"=w661, "BG Color"=w660) -> ()  [unwired: 2 in, 2 out]
          "Trigger histogram 31" <- w662
        }
        frame 32 {
          n258 = property on="Trigger histogram 32" class="XYGraph (strict)"("TipStrip"=w664, "BG Color"=w663) -> ()  [unwired: 2 in, 2 out]
          "Trigger histogram 32" <- w665
        }
        frame 33 {
          n259 = property on="Trigger histogram 33" class="XYGraph (strict)"("TipStrip"=w667, "BG Color"=w666) -> ()  [unwired: 2 in, 2 out]
          "Trigger histogram 33" <- w668
        }
        frame 34 {
          n260 = property on="Trigger histogram 34" class="XYGraph (strict)"("TipStrip"=w670, "BG Color"=w669) -> ()  [unwired: 2 in, 2 out]
          "Trigger histogram 34" <- w671
        }
        frame 35 {
          n261 = property on="Trigger histogram 35" class="XYGraph (strict)"("TipStrip"=w673, "BG Color"=w672) -> ()  [unwired: 2 in, 2 out]
          "Trigger histogram 35" <- w674
        }
        frame 36 {
          n262 = property on="Trigger histogram 36" class="XYGraph (strict)"("TipStrip"=w676, "BG Color"=w675) -> ()  [unwired: 2 in, 2 out]
          "Trigger histogram 36" <- w677
        }
        frame 37 {
          n263 = property on="Trigger histogram 37" class="XYGraph (strict)"("TipStrip"=w679, "BG Color"=w678) -> ()  [unwired: 2 in, 2 out]
          "Trigger histogram 37" <- w680
        }
        frame 38 {
          n264 = property on="Trigger histogram 38" class="XYGraph (strict)"("TipStrip"=w682, "BG Color"=w681) -> ()  [unwired: 2 in, 2 out]
          "Trigger histogram 38" <- w683
        }
        frame 39 {
          n265 = property on="Trigger histogram 39" class="XYGraph (strict)"("TipStrip"=w685, "BG Color"=w684) -> ()  [unwired: 2 in, 2 out]
          "Trigger histogram 39" <- w686
        }
        frame 40 {
          n266 = property on="Trigger histogram 40" class="XYGraph (strict)"("TipStrip"=w688, "BG Color"=w687) -> ()  [unwired: 2 in, 2 out]
          "Trigger histogram 40" <- w689
        }
        frame 41 {
          n267 = property on="Trigger histogram 41" class="XYGraph (strict)"("TipStrip"=w691, "BG Color"=w690) -> ()  [unwired: 2 in, 2 out]
          "Trigger histogram 41" <- w692
        }
        frame 42 {
          n268 = property on="Trigger histogram 42" class="XYGraph (strict)"("TipStrip"=w694, "BG Color"=w693) -> ()  [unwired: 2 in, 2 out]
          "Trigger histogram 42" <- w695
        }
        frame 43 {
          n269 = property on="Trigger histogram 43" class="XYGraph (strict)"("TipStrip"=w697, "BG Color"=w696) -> ()  [unwired: 2 in, 2 out]
          "Trigger histogram 43" <- w698
        }
        frame 44 {
          n270 = property on="Trigger histogram 44" class="XYGraph (strict)"("TipStrip"=w700, "BG Color"=w699) -> ()  [unwired: 2 in, 2 out]
          "Trigger histogram 44" <- w701
        }
        frame 45 {
          n271 = property on="Trigger histogram 45" class="XYGraph (strict)"("TipStrip"=w703, "BG Color"=w702) -> ()  [unwired: 2 in, 2 out]
          "Trigger histogram 45" <- w704
        }
        frame 46 {
          n272 = property on="Trigger histogram 46" class="XYGraph (strict)"("TipStrip"=w706, "BG Color"=w705) -> ()  [unwired: 2 in, 2 out]
          "Trigger histogram 46" <- w707
        }
        frame 47 {
          n273 = property on="Trigger histogram 47" class="XYGraph (strict)"("TipStrip"=w709, "BG Color"=w708) -> ()  [unwired: 2 in, 2 out]
          "Trigger histogram 47" <- w710
        }
        frame 48 {
          n274 = property on="Trigger histogram 48" class="XYGraph (strict)"("TipStrip"=w712, "BG Color"=w711) -> ()  [unwired: 2 in, 2 out]
          "Trigger histogram 48" <- w713
        }
        frame 49 {
          n275 = property on="Trigger histogram 49" class="XYGraph (strict)"("TipStrip"=w715, "BG Color"=w714) -> ()  [unwired: 2 in, 2 out]
          "Trigger histogram 49" <- w716
        }
        frame 50 {
          n276 = property on="Trigger histogram 50" class="XYGraph (strict)"("TipStrip"=w718, "BG Color"=w717) -> ()  [unwired: 2 in, 2 out]
          "Trigger histogram 50" <- w719
        }
        frame 51 {
          n277 = property on="Trigger histogram 51" class="XYGraph (strict)"("TipStrip"=w721, "BG Color"=w720) -> ()  [unwired: 2 in, 2 out]
          "Trigger histogram 51" <- w722
        }
        frame 52 {
          n278 = property on="Trigger histogram 52" class="XYGraph (strict)"("TipStrip"=w724, "BG Color"=w723) -> ()  [unwired: 2 in, 2 out]
          "Trigger histogram 52" <- w725
        }
        frame 53 {
          n279 = property on="Trigger histogram 53" class="XYGraph (strict)"("TipStrip"=w727, "BG Color"=w726) -> ()  [unwired: 2 in, 2 out]
          "Trigger histogram 53" <- w728
        }
        frame 54 {
          n280 = property on="Trigger histogram 54" class="XYGraph (strict)"("TipStrip"=w730, "BG Color"=w729) -> ()  [unwired: 2 in, 2 out]
          "Trigger histogram 54" <- w731
        }
        frame 55 {
          n281 = property on="Trigger histogram 55" class="XYGraph (strict)"("TipStrip"=w733, "BG Color"=w732) -> ()  [unwired: 2 in, 2 out]
          "Trigger histogram 55" <- w734
        }
        frame 56 {
          n282 = property on="Trigger histogram 56" class="XYGraph (strict)"("TipStrip"=w736, "BG Color"=w735) -> ()  [unwired: 2 in, 2 out]
          "Trigger histogram 56" <- w737
        }
        frame 57 {
          n283 = property on="Trigger histogram 57" class="XYGraph (strict)"("TipStrip"=w739, "BG Color"=w738) -> ()  [unwired: 2 in, 2 out]
          "Trigger histogram 57" <- w740
        }
        frame 58 {
          n284 = property on="Trigger histogram 58" class="XYGraph (strict)"("TipStrip"=w742, "BG Color"=w741) -> ()  [unwired: 2 in, 2 out]
          "Trigger histogram 58" <- w743
        }
        frame 59 {
          n285 = property on="Trigger histogram 59" class="XYGraph (strict)"("TipStrip"=w745, "BG Color"=w744) -> ()  [unwired: 2 in, 2 out]
          "Trigger histogram 59" <- w746
        }
        frame 60 {
          n286 = property on="Trigger histogram 60" class="XYGraph (strict)"("TipStrip"=w748, "BG Color"=w747) -> ()  [unwired: 2 in, 2 out]
          "Trigger histogram 60" <- w749
        }
        frame 61 {
          n287 = property on="Trigger histogram 61" class="XYGraph (strict)"("TipStrip"=w751, "BG Color"=w750) -> ()  [unwired: 2 in, 2 out]
          "Trigger histogram 61" <- w752
        }
        frame 62 {
          n288 = property on="Trigger histogram 62" class="XYGraph (strict)"("TipStrip"=w754, "BG Color"=w753) -> ()  [unwired: 2 in, 2 out]
          "Trigger histogram 62" <- w755
        }
        frame 63 {
          n289 = property on="Trigger histogram 63" class="XYGraph (strict)"("TipStrip"=w757, "BG Color"=w756) -> ()  [unwired: 2 in, 2 out]
          "Trigger histogram 63" <- w758
        }
        frame 64 {
          n290 = property on="Trigger histogram 64" class="XYGraph (strict)"("TipStrip"=w760, "BG Color"=w759) -> ()  [unwired: 2 in, 2 out]
          "Trigger histogram 64" <- w761
        }
        frame 65 {
          n291 = property on="Trigger histogram 65" class="XYGraph (strict)"("TipStrip"=w763, "BG Color"=w762) -> ()  [unwired: 2 in, 2 out]
          "Trigger histogram 65" <- w764
        }
        frame 66 {
          n292 = property on="Trigger histogram 66" class="XYGraph (strict)"("TipStrip"=w766, "BG Color"=w765) -> ()  [unwired: 2 in, 2 out]
          "Trigger histogram 66" <- w767
        }
        frame 67 {
          n293 = property on="Trigger histogram 67" class="XYGraph (strict)"("TipStrip"=w769, "BG Color"=w768) -> ()  [unwired: 2 in, 2 out]
          "Trigger histogram 67" <- w770
        }
        frame 68 {
          n294 = property on="Trigger histogram 68" class="XYGraph (strict)"("TipStrip"=w772, "BG Color"=w771) -> ()  [unwired: 2 in, 2 out]
          "Trigger histogram 68" <- w773
        }
        frame 69 {
          n295 = property on="Trigger histogram 69" class="XYGraph (strict)"("TipStrip"=w775, "BG Color"=w774) -> ()  [unwired: 2 in, 2 out]
          "Trigger histogram 69" <- w776
        }
        frame 70 {
          n296 = property on="Trigger histogram 70" class="XYGraph (strict)"("TipStrip"=w778, "BG Color"=w777) -> ()  [unwired: 2 in, 2 out]
          "Trigger histogram 70" <- w779
        }
        frame 71 {
          n297 = property on="Trigger histogram 71" class="XYGraph (strict)"("TipStrip"=w781, "BG Color"=w780) -> ()  [unwired: 2 in, 2 out]
          "Trigger histogram 71" <- w782
        }
        frame 72 {
          n298 = property on="Trigger histogram 72" class="XYGraph (strict)"("TipStrip"=w784, "BG Color"=w783) -> ()  [unwired: 2 in, 2 out]
          "Trigger histogram 72" <- w785
        }
        frame 73 {
          n299 = property on="Trigger histogram 73" class="XYGraph (strict)"("TipStrip"=w787, "BG Color"=w786) -> ()  [unwired: 2 in, 2 out]
          "Trigger histogram 73" <- w788
        }
        frame 74 {
          n300 = property on="Trigger histogram 74" class="XYGraph (strict)"("TipStrip"=w790, "BG Color"=w789) -> ()  [unwired: 2 in, 2 out]
          "Trigger histogram 74" <- w791
        }
        frame 75 {
          n301 = property on="Trigger histogram 75" class="XYGraph (strict)"("TipStrip"=w793, "BG Color"=w792) -> ()  [unwired: 2 in, 2 out]
          "Trigger histogram 75" <- w794
        }
        frame 76 {
          n302 = property on="Trigger histogram 76" class="XYGraph (strict)"("TipStrip"=w796, "BG Color"=w795) -> ()  [unwired: 2 in, 2 out]
          "Trigger histogram 76" <- w797
        }
        frame 77 {
          n303 = property on="Trigger histogram 77" class="XYGraph (strict)"("TipStrip"=w799, "BG Color"=w798) -> ()  [unwired: 2 in, 2 out]
          "Trigger histogram 77" <- w800
        }
        frame 78 {
          n304 = property on="Trigger histogram 78" class="XYGraph (strict)"("TipStrip"=w802, "BG Color"=w801) -> ()  [unwired: 2 in, 2 out]
          "Trigger histogram 78" <- w803
        }
        frame 79 {
          n305 = property on="Trigger histogram 79" class="XYGraph (strict)"("TipStrip"=w805, "BG Color"=w804) -> ()  [unwired: 2 in, 2 out]
          "Trigger histogram 79" <- w806
        }
        frame 80 {
          n306 = property on="Trigger histogram 80" class="XYGraph (strict)"("TipStrip"=w808, "BG Color"=w807) -> ()  [unwired: 2 in, 2 out]
          "Trigger histogram 80" <- w809
        }
        frame 81 {
          n307 = property on="Trigger histogram 81" class="XYGraph (strict)"("TipStrip"=w811, "BG Color"=w810) -> ()  [unwired: 2 in, 2 out]
          "Trigger histogram 81" <- w812
        }
        frame 82 {
          n308 = property on="Trigger histogram 82" class="XYGraph (strict)"("TipStrip"=w814, "BG Color"=w813) -> ()  [unwired: 2 in, 2 out]
          "Trigger histogram 82" <- w815
        }
        frame 83 {
          n309 = property on="Trigger histogram 83" class="XYGraph (strict)"("TipStrip"=w817, "BG Color"=w816) -> ()  [unwired: 2 in, 2 out]
          "Trigger histogram 83" <- w818
        }
        frame 84 {
          n310 = property on="Trigger histogram 84" class="XYGraph (strict)"("TipStrip"=w820, "BG Color"=w819) -> ()  [unwired: 2 in, 2 out]
          "Trigger histogram 84" <- w821
        }
        frame 85 {
          n311 = property on="Trigger histogram 85" class="XYGraph (strict)"("TipStrip"=w823, "BG Color"=w822) -> ()  [unwired: 2 in, 2 out]
          "Trigger histogram 85" <- w824
        }
        frame 86 {
          n312 = property on="Trigger histogram 86" class="XYGraph (strict)"("TipStrip"=w826, "BG Color"=w825) -> ()  [unwired: 2 in, 2 out]
          "Trigger histogram 86" <- w827
        }
        frame 87 {
          n313 = property on="Trigger histogram 87" class="XYGraph (strict)"("TipStrip"=w829, "BG Color"=w828) -> ()  [unwired: 2 in, 2 out]
          "Trigger histogram 87" <- w830
        }
        frame 88 {
          n314 = property on="Trigger histogram 88" class="XYGraph (strict)"("TipStrip"=w832, "BG Color"=w831) -> ()  [unwired: 2 in, 2 out]
          "Trigger histogram 88" <- w833
        }
        frame 89 {
          n315 = property on="Trigger histogram 89" class="XYGraph (strict)"("TipStrip"=w835, "BG Color"=w834) -> ()  [unwired: 2 in, 2 out]
          "Trigger histogram 89" <- w836
        }
        frame 90 {
          n316 = property on="Trigger histogram 90" class="XYGraph (strict)"("TipStrip"=w838, "BG Color"=w837) -> ()  [unwired: 2 in, 2 out]
          "Trigger histogram 90" <- w839
        }
        frame 91 {
          n317 = property on="Trigger histogram 91" class="XYGraph (strict)"("TipStrip"=w841, "BG Color"=w840) -> ()  [unwired: 2 in, 2 out]
          "Trigger histogram 91" <- w842
        }
        frame 92 {
          n318 = property on="Trigger histogram 92" class="XYGraph (strict)"("TipStrip"=w844, "BG Color"=w843) -> ()  [unwired: 2 in, 2 out]
          "Trigger histogram 92" <- w845
        }
        frame 93 {
          n319 = property on="Trigger histogram 93" class="XYGraph (strict)"("TipStrip"=w847, "BG Color"=w846) -> ()  [unwired: 2 in, 2 out]
          "Trigger histogram 93" <- w848
        }
        frame 94 {
          n320 = property on="Trigger histogram 94" class="XYGraph (strict)"("TipStrip"=w850, "BG Color"=w849) -> ()  [unwired: 2 in, 2 out]
          "Trigger histogram 94" <- w851
        }
        frame 95 {
          n321 = property on="Trigger histogram 95" class="XYGraph (strict)"("TipStrip"=w853, "BG Color"=w852) -> ()  [unwired: 2 in, 2 out]
          "Trigger histogram 95" <- w854
        }
        frame 96 {
          n322 = property on="Trigger histogram 96" class="XYGraph (strict)"("TipStrip"=w856, "BG Color"=w855) -> ()  [unwired: 2 in, 2 out]
          "Trigger histogram 96" <- w857
        }
        frame 97 {
          n323 = property on="Trigger histogram 97" class="XYGraph (strict)"("TipStrip"=w859, "BG Color"=w858) -> ()  [unwired: 2 in, 2 out]
          "Trigger histogram 97" <- w860
        }
        frame 98 {
          n324 = property on="Trigger histogram 98" class="XYGraph (strict)"("TipStrip"=w862, "BG Color"=w861) -> ()  [unwired: 2 in, 2 out]
          "Trigger histogram 98" <- w863
        }
        frame 99 {
          n325 = property on="Trigger histogram 99" class="XYGraph (strict)"("TipStrip"=w865, "BG Color"=w864) -> ()  [unwired: 2 in, 2 out]
          "Trigger histogram 99" <- w866
        }
      }
    }
    n326 = flat-sequence {
      tunnel: w165 -> [w215]
      tunnel: [w216] -> w164
      frame #0 {
        "Total number of events" <- w215
      }
      frame #1 {
        # "User interactions: buttons"
        n327 = while {
          tunnel: [w218] -> w216
          stop <- w217 stop-if-true
          n328 = event shown="[3] \"Y scale\", \"X scale min.\", \"X scale max.\": Value Change" {
            selector: _ -> [_ _ _ _ _]
            dyn-events: _ -> [_ _ _ _ _]
            timeout: _ -> [_ _ _ _ _]
            tunnel: [_ w219 w221 w226 w531] -> w218
            tunnel: [_ w219 TRUE ("Close viewer") w226 w531] -> w217
            event Timeout {
              n329 = event-data() -> ()  [unwired: 1 in, 2 out]
            }
            event "Close button": Value Change {
              w219 = TRUE  # Close viewer
              n330 = event-data() -> ()  [unwired: 1 in, 6 out]
            }
            event "Choose Chip button": Mouse Down {
              w221 = FALSE  # Another iteration: choose ChipID
              n331 = event-data() -> ()  [unwired: 1 in, 7 out]
            }
            event "Y scale", "X scale min.", "X scale max.": Value Change {
              w226 = FALSE ("Close viewer")
              n332 = event-data() -> ()  [unwired: 1 in, 5 out]
              n333 = for {
                N: 100 -> [_]
                tunnel: "Y scale" -> [w229]
                tunnel: "X scale min." -> [w228]
                tunnel: "X scale max." -> [w227]
                i -> [w230]
                # "Fix Scales"
                n334 = case shown="0" w230 {
                  tunnel: w229 -> [_ w233 w236 w239 w242 w245 w248 w251 w254 w257 w260 w263 w266 w269 w272 w275 w278 w281 w284 w287 w290 w293 w296 w299 w302 w305 w308 w311 w314 w317 w320 w323 w326 w329 w332 w335 w338 w341 w344 w347 w350 w353 w356 w359 w362 w365 w368 w371 w374 w377 w380 w383 w386 w389 w392 w395 w398 w401 w404 w407 w410 w413 w416 w419 w422 w425 w428 w431 w434 w437 w440 w443 w446 w449 w452 w455 w458 w461 w464 w467 w470 w473 w476 w479 w482 w485 w488 w491 w494 w497 w500 w503 w506 w509 w512 w515 w518 w521 w524 w527 w530]
                  tunnel: w228 -> [_ w232 w235 w238 w241 w244 w247 w250 w253 w256 w259 w262 w265 w268 w271 w274 w277 w280 w283 w286 w289 w292 w295 w298 w301 w304 w307 w310 w313 w316 w319 w322 w325 w328 w331 w334 w337 w340 w343 w346 w349 w352 w355 w358 w361 w364 w367 w370 w373 w376 w379 w382 w385 w388 w391 w394 w397 w400 w403 w406 w409 w412 w415 w418 w421 w424 w427 w430 w433 w436 w439 w442 w445 w448 w451 w454 w457 w460 w463 w466 w469 w472 w475 w478 w481 w484 w487 w490 w493 w496 w499 w502 w505 w508 w511 w514 w517 w520 w523 w526 w529]
                  tunnel: w227 -> [_ w231 w234 w237 w240 w243 w246 w249 w252 w255 w258 w261 w264 w267 w270 w273 w276 w279 w282 w285 w288 w291 w294 w297 w300 w303 w306 w309 w312 w315 w318 w321 w324 w327 w330 w333 w336 w339 w342 w345 w348 w351 w354 w357 w360 w363 w366 w369 w372 w375 w378 w381 w384 w387 w390 w393 w396 w399 w402 w405 w408 w411 w414 w417 w420 w423 w426 w429 w432 w435 w438 w441 w444 w447 w450 w453 w456 w459 w462 w465 w468 w471 w474 w477 w480 w483 w486 w489 w492 w495 w498 w501 w504 w507 w510 w513 w516 w519 w522 w525 w528]
                  frame Default {
                  }
                  frame 0 {
                    n335 = property on="Trigger histogram 00" class="XYGraph (strict)"("YScale.Maximum"=w233, "XScale.Minimum"=w232, "XScale.Maximum"=w231) -> ()  [unwired: 2 in, 2 out]
                  }
                  frame 1 {
                    n336 = property on="Trigger histogram 01" class="XYGraph (strict)"("YScale.Maximum"=w236, "XScale.Minimum"=w235, "XScale.Maximum"=w234) -> ()  [unwired: 2 in, 2 out]
                  }
                  frame 2 {
                    n337 = property on="Trigger histogram 02" class="XYGraph (strict)"("YScale.Maximum"=w239, "XScale.Minimum"=w238, "XScale.Maximum"=w237) -> ()  [unwired: 2 in, 2 out]
                  }
                  frame 3 {
                    n338 = property on="Trigger histogram 03" class="XYGraph (strict)"("YScale.Maximum"=w242, "XScale.Minimum"=w241, "XScale.Maximum"=w240) -> ()  [unwired: 2 in, 2 out]
                  }
                  frame 4 {
                    n339 = property on="Trigger histogram 04" class="XYGraph (strict)"("YScale.Maximum"=w245, "XScale.Minimum"=w244, "XScale.Maximum"=w243) -> ()  [unwired: 2 in, 2 out]
                  }
                  frame 5 {
                    n340 = property on="Trigger histogram 05" class="XYGraph (strict)"("YScale.Maximum"=w248, "XScale.Minimum"=w247, "XScale.Maximum"=w246) -> ()  [unwired: 2 in, 2 out]
                  }
                  frame 6 {
                    n341 = property on="Trigger histogram 06" class="XYGraph (strict)"("YScale.Maximum"=w251, "XScale.Minimum"=w250, "XScale.Maximum"=w249) -> ()  [unwired: 2 in, 2 out]
                  }
                  frame 7 {
                    n342 = property on="Trigger histogram 07" class="XYGraph (strict)"("YScale.Maximum"=w254, "XScale.Minimum"=w253, "XScale.Maximum"=w252) -> ()  [unwired: 2 in, 2 out]
                  }
                  frame 8 {
                    n343 = property on="Trigger histogram 08" class="XYGraph (strict)"("YScale.Maximum"=w257, "XScale.Minimum"=w256, "XScale.Maximum"=w255) -> ()  [unwired: 2 in, 2 out]
                  }
                  frame 9 {
                    n344 = property on="Trigger histogram 09" class="XYGraph (strict)"("YScale.Maximum"=w260, "XScale.Minimum"=w259, "XScale.Maximum"=w258) -> ()  [unwired: 2 in, 2 out]
                  }
                  frame 10 {
                    n345 = property on="Trigger histogram 10" class="XYGraph (strict)"("YScale.Maximum"=w263, "XScale.Minimum"=w262, "XScale.Maximum"=w261) -> ()  [unwired: 2 in, 2 out]
                  }
                  frame 11 {
                    n346 = property on="Trigger histogram 11" class="XYGraph (strict)"("YScale.Maximum"=w266, "XScale.Minimum"=w265, "XScale.Maximum"=w264) -> ()  [unwired: 2 in, 2 out]
                  }
                  frame 12 {
                    n347 = property on="Trigger histogram 12" class="XYGraph (strict)"("YScale.Maximum"=w269, "XScale.Minimum"=w268, "XScale.Maximum"=w267) -> ()  [unwired: 2 in, 2 out]
                  }
                  frame 13 {
                    n348 = property on="Trigger histogram 13" class="XYGraph (strict)"("YScale.Maximum"=w272, "XScale.Minimum"=w271, "XScale.Maximum"=w270) -> ()  [unwired: 2 in, 2 out]
                  }
                  frame 14 {
                    n349 = property on="Trigger histogram 14" class="XYGraph (strict)"("YScale.Maximum"=w275, "XScale.Minimum"=w274, "XScale.Maximum"=w273) -> ()  [unwired: 2 in, 2 out]
                  }
                  frame 15 {
                    n350 = property on="Trigger histogram 15" class="XYGraph (strict)"("YScale.Maximum"=w278, "XScale.Minimum"=w277, "XScale.Maximum"=w276) -> ()  [unwired: 2 in, 2 out]
                  }
                  frame 16 {
                    n351 = property on="Trigger histogram 16" class="XYGraph (strict)"("YScale.Maximum"=w281, "XScale.Minimum"=w280, "XScale.Maximum"=w279) -> ()  [unwired: 2 in, 2 out]
                  }
                  frame 17 {
                    n352 = property on="Trigger histogram 17" class="XYGraph (strict)"("YScale.Maximum"=w284, "XScale.Minimum"=w283, "XScale.Maximum"=w282) -> ()  [unwired: 2 in, 2 out]
                  }
                  frame 18 {
                    n353 = property on="Trigger histogram 18" class="XYGraph (strict)"("YScale.Maximum"=w287, "XScale.Minimum"=w286, "XScale.Maximum"=w285) -> ()  [unwired: 2 in, 2 out]
                  }
                  frame 19 {
                    n354 = property on="Trigger histogram 19" class="XYGraph (strict)"("YScale.Maximum"=w290, "XScale.Minimum"=w289, "XScale.Maximum"=w288) -> ()  [unwired: 2 in, 2 out]
                  }
                  frame 20 {
                    n355 = property on="Trigger histogram 20" class="XYGraph (strict)"("YScale.Maximum"=w293, "XScale.Minimum"=w292, "XScale.Maximum"=w291) -> ()  [unwired: 2 in, 2 out]
                  }
                  frame 21 {
                    n356 = property on="Trigger histogram 21" class="XYGraph (strict)"("YScale.Maximum"=w296, "XScale.Minimum"=w295, "XScale.Maximum"=w294) -> ()  [unwired: 2 in, 2 out]
                  }
                  frame 22 {
                    n357 = property on="Trigger histogram 22" class="XYGraph (strict)"("YScale.Maximum"=w299, "XScale.Minimum"=w298, "XScale.Maximum"=w297) -> ()  [unwired: 2 in, 2 out]
                  }
                  frame 23 {
                    n358 = property on="Trigger histogram 23" class="XYGraph (strict)"("YScale.Maximum"=w302, "XScale.Minimum"=w301, "XScale.Maximum"=w300) -> ()  [unwired: 2 in, 2 out]
                  }
                  frame 24 {
                    n359 = property on="Trigger histogram 24" class="XYGraph (strict)"("YScale.Maximum"=w305, "XScale.Minimum"=w304, "XScale.Maximum"=w303) -> ()  [unwired: 2 in, 2 out]
                  }
                  frame 25 {
                    n360 = property on="Trigger histogram 25" class="XYGraph (strict)"("YScale.Maximum"=w308, "XScale.Minimum"=w307, "XScale.Maximum"=w306) -> ()  [unwired: 2 in, 2 out]
                  }
                  frame 26 {
                    n361 = property on="Trigger histogram 26" class="XYGraph (strict)"("YScale.Maximum"=w311, "XScale.Minimum"=w310, "XScale.Maximum"=w309) -> ()  [unwired: 2 in, 2 out]
                  }
                  frame 27 {
                    n362 = property on="Trigger histogram 27" class="XYGraph (strict)"("YScale.Maximum"=w314, "XScale.Minimum"=w313, "XScale.Maximum"=w312) -> ()  [unwired: 2 in, 2 out]
                  }
                  frame 28 {
                    n363 = property on="Trigger histogram 28" class="XYGraph (strict)"("YScale.Maximum"=w317, "XScale.Minimum"=w316, "XScale.Maximum"=w315) -> ()  [unwired: 2 in, 2 out]
                  }
                  frame 29 {
                    n364 = property on="Trigger histogram 29" class="XYGraph (strict)"("YScale.Maximum"=w320, "XScale.Minimum"=w319, "XScale.Maximum"=w318) -> ()  [unwired: 2 in, 2 out]
                  }
                  frame 30 {
                    n365 = property on="Trigger histogram 30" class="XYGraph (strict)"("YScale.Maximum"=w323, "XScale.Minimum"=w322, "XScale.Maximum"=w321) -> ()  [unwired: 2 in, 2 out]
                  }
                  frame 31 {
                    n366 = property on="Trigger histogram 31" class="XYGraph (strict)"("YScale.Maximum"=w326, "XScale.Minimum"=w325, "XScale.Maximum"=w324) -> ()  [unwired: 2 in, 2 out]
                  }
                  frame 32 {
                    n367 = property on="Trigger histogram 32" class="XYGraph (strict)"("YScale.Maximum"=w329, "XScale.Minimum"=w328, "XScale.Maximum"=w327) -> ()  [unwired: 2 in, 2 out]
                  }
                  frame 33 {
                    n368 = property on="Trigger histogram 33" class="XYGraph (strict)"("YScale.Maximum"=w332, "XScale.Minimum"=w331, "XScale.Maximum"=w330) -> ()  [unwired: 2 in, 2 out]
                  }
                  frame 34 {
                    n369 = property on="Trigger histogram 34" class="XYGraph (strict)"("YScale.Maximum"=w335, "XScale.Minimum"=w334, "XScale.Maximum"=w333) -> ()  [unwired: 2 in, 2 out]
                  }
                  frame 35 {
                    n370 = property on="Trigger histogram 35" class="XYGraph (strict)"("YScale.Maximum"=w338, "XScale.Minimum"=w337, "XScale.Maximum"=w336) -> ()  [unwired: 2 in, 2 out]
                  }
                  frame 36 {
                    n371 = property on="Trigger histogram 36" class="XYGraph (strict)"("YScale.Maximum"=w341, "XScale.Minimum"=w340, "XScale.Maximum"=w339) -> ()  [unwired: 2 in, 2 out]
                  }
                  frame 37 {
                    n372 = property on="Trigger histogram 37" class="XYGraph (strict)"("YScale.Maximum"=w344, "XScale.Minimum"=w343, "XScale.Maximum"=w342) -> ()  [unwired: 2 in, 2 out]
                  }
                  frame 38 {
                    n373 = property on="Trigger histogram 38" class="XYGraph (strict)"("YScale.Maximum"=w347, "XScale.Minimum"=w346, "XScale.Maximum"=w345) -> ()  [unwired: 2 in, 2 out]
                  }
                  frame 39 {
                    n374 = property on="Trigger histogram 39" class="XYGraph (strict)"("YScale.Maximum"=w350, "XScale.Minimum"=w349, "XScale.Maximum"=w348) -> ()  [unwired: 2 in, 2 out]
                  }
                  frame 40 {
                    n375 = property on="Trigger histogram 40" class="XYGraph (strict)"("YScale.Maximum"=w353, "XScale.Minimum"=w352, "XScale.Maximum"=w351) -> ()  [unwired: 2 in, 2 out]
                  }
                  frame 41 {
                    n376 = property on="Trigger histogram 41" class="XYGraph (strict)"("YScale.Maximum"=w356, "XScale.Minimum"=w355, "XScale.Maximum"=w354) -> ()  [unwired: 2 in, 2 out]
                  }
                  frame 42 {
                    n377 = property on="Trigger histogram 42" class="XYGraph (strict)"("YScale.Maximum"=w359, "XScale.Minimum"=w358, "XScale.Maximum"=w357) -> ()  [unwired: 2 in, 2 out]
                  }
                  frame 43 {
                    n378 = property on="Trigger histogram 43" class="XYGraph (strict)"("YScale.Maximum"=w362, "XScale.Minimum"=w361, "XScale.Maximum"=w360) -> ()  [unwired: 2 in, 2 out]
                  }
                  frame 44 {
                    n379 = property on="Trigger histogram 44" class="XYGraph (strict)"("YScale.Maximum"=w365, "XScale.Minimum"=w364, "XScale.Maximum"=w363) -> ()  [unwired: 2 in, 2 out]
                  }
                  frame 45 {
                    n380 = property on="Trigger histogram 45" class="XYGraph (strict)"("YScale.Maximum"=w368, "XScale.Minimum"=w367, "XScale.Maximum"=w366) -> ()  [unwired: 2 in, 2 out]
                  }
                  frame 46 {
                    n381 = property on="Trigger histogram 46" class="XYGraph (strict)"("YScale.Maximum"=w371, "XScale.Minimum"=w370, "XScale.Maximum"=w369) -> ()  [unwired: 2 in, 2 out]
                  }
                  frame 47 {
                    n382 = property on="Trigger histogram 47" class="XYGraph (strict)"("YScale.Maximum"=w374, "XScale.Minimum"=w373, "XScale.Maximum"=w372) -> ()  [unwired: 2 in, 2 out]
                  }
                  frame 48 {
                    n383 = property on="Trigger histogram 48" class="XYGraph (strict)"("YScale.Maximum"=w377, "XScale.Minimum"=w376, "XScale.Maximum"=w375) -> ()  [unwired: 2 in, 2 out]
                  }
                  frame 49 {
                    n384 = property on="Trigger histogram 49" class="XYGraph (strict)"("YScale.Maximum"=w380, "XScale.Minimum"=w379, "XScale.Maximum"=w378) -> ()  [unwired: 2 in, 2 out]
                  }
                  frame 50 {
                    n385 = property on="Trigger histogram 50" class="XYGraph (strict)"("YScale.Maximum"=w383, "XScale.Minimum"=w382, "XScale.Maximum"=w381) -> ()  [unwired: 2 in, 2 out]
                  }
                  frame 51 {
                    n386 = property on="Trigger histogram 51" class="XYGraph (strict)"("YScale.Maximum"=w386, "XScale.Minimum"=w385, "XScale.Maximum"=w384) -> ()  [unwired: 2 in, 2 out]
                  }
                  frame 52 {
                    n387 = property on="Trigger histogram 52" class="XYGraph (strict)"("YScale.Maximum"=w389, "XScale.Minimum"=w388, "XScale.Maximum"=w387) -> ()  [unwired: 2 in, 2 out]
                  }
                  frame 53 {
                    n388 = property on="Trigger histogram 53" class="XYGraph (strict)"("YScale.Maximum"=w392, "XScale.Minimum"=w391, "XScale.Maximum"=w390) -> ()  [unwired: 2 in, 2 out]
                  }
                  frame 54 {
                    n389 = property on="Trigger histogram 54" class="XYGraph (strict)"("YScale.Maximum"=w395, "XScale.Minimum"=w394, "XScale.Maximum"=w393) -> ()  [unwired: 2 in, 2 out]
                  }
                  frame 55 {
                    n390 = property on="Trigger histogram 55" class="XYGraph (strict)"("YScale.Maximum"=w398, "XScale.Minimum"=w397, "XScale.Maximum"=w396) -> ()  [unwired: 2 in, 2 out]
                  }
                  frame 56 {
                    n391 = property on="Trigger histogram 56" class="XYGraph (strict)"("YScale.Maximum"=w401, "XScale.Minimum"=w400, "XScale.Maximum"=w399) -> ()  [unwired: 2 in, 2 out]
                  }
                  frame 57 {
                    n392 = property on="Trigger histogram 57" class="XYGraph (strict)"("YScale.Maximum"=w404, "XScale.Minimum"=w403, "XScale.Maximum"=w402) -> ()  [unwired: 2 in, 2 out]
                  }
                  frame 58 {
                    n393 = property on="Trigger histogram 58" class="XYGraph (strict)"("YScale.Maximum"=w407, "XScale.Minimum"=w406, "XScale.Maximum"=w405) -> ()  [unwired: 2 in, 2 out]
                  }
                  frame 59 {
                    n394 = property on="Trigger histogram 59" class="XYGraph (strict)"("YScale.Maximum"=w410, "XScale.Minimum"=w409, "XScale.Maximum"=w408) -> ()  [unwired: 2 in, 2 out]
                  }
                  frame 60 {
                    n395 = property on="Trigger histogram 60" class="XYGraph (strict)"("YScale.Maximum"=w413, "XScale.Minimum"=w412, "XScale.Maximum"=w411) -> ()  [unwired: 2 in, 2 out]
                  }
                  frame 61 {
                    n396 = property on="Trigger histogram 61" class="XYGraph (strict)"("YScale.Maximum"=w416, "XScale.Minimum"=w415, "XScale.Maximum"=w414) -> ()  [unwired: 2 in, 2 out]
                  }
                  frame 62 {
                    n397 = property on="Trigger histogram 62" class="XYGraph (strict)"("YScale.Maximum"=w419, "XScale.Minimum"=w418, "XScale.Maximum"=w417) -> ()  [unwired: 2 in, 2 out]
                  }
                  frame 63 {
                    n398 = property on="Trigger histogram 63" class="XYGraph (strict)"("YScale.Maximum"=w422, "XScale.Minimum"=w421, "XScale.Maximum"=w420) -> ()  [unwired: 2 in, 2 out]
                  }
                  frame 64 {
                    n399 = property on="Trigger histogram 64" class="XYGraph (strict)"("YScale.Maximum"=w425, "XScale.Minimum"=w424, "XScale.Maximum"=w423) -> ()  [unwired: 2 in, 2 out]
                  }
                  frame 65 {
                    n400 = property on="Trigger histogram 65" class="XYGraph (strict)"("YScale.Maximum"=w428, "XScale.Minimum"=w427, "XScale.Maximum"=w426) -> ()  [unwired: 2 in, 2 out]
                  }
                  frame 66 {
                    n401 = property on="Trigger histogram 66" class="XYGraph (strict)"("YScale.Maximum"=w431, "XScale.Minimum"=w430, "XScale.Maximum"=w429) -> ()  [unwired: 2 in, 2 out]
                  }
                  frame 67 {
                    n402 = property on="Trigger histogram 67" class="XYGraph (strict)"("YScale.Maximum"=w434, "XScale.Minimum"=w433, "XScale.Maximum"=w432) -> ()  [unwired: 2 in, 2 out]
                  }
                  frame 68 {
                    n403 = property on="Trigger histogram 68" class="XYGraph (strict)"("YScale.Maximum"=w437, "XScale.Minimum"=w436, "XScale.Maximum"=w435) -> ()  [unwired: 2 in, 2 out]
                  }
                  frame 69 {
                    n404 = property on="Trigger histogram 69" class="XYGraph (strict)"("YScale.Maximum"=w440, "XScale.Minimum"=w439, "XScale.Maximum"=w438) -> ()  [unwired: 2 in, 2 out]
                  }
                  frame 70 {
                    n405 = property on="Trigger histogram 70" class="XYGraph (strict)"("YScale.Maximum"=w443, "XScale.Minimum"=w442, "XScale.Maximum"=w441) -> ()  [unwired: 2 in, 2 out]
                  }
                  frame 71 {
                    n406 = property on="Trigger histogram 71" class="XYGraph (strict)"("YScale.Maximum"=w446, "XScale.Minimum"=w445, "XScale.Maximum"=w444) -> ()  [unwired: 2 in, 2 out]
                  }
                  frame 72 {
                    n407 = property on="Trigger histogram 72" class="XYGraph (strict)"("YScale.Maximum"=w449, "XScale.Minimum"=w448, "XScale.Maximum"=w447) -> ()  [unwired: 2 in, 2 out]
                  }
                  frame 73 {
                    n408 = property on="Trigger histogram 73" class="XYGraph (strict)"("YScale.Maximum"=w452, "XScale.Minimum"=w451, "XScale.Maximum"=w450) -> ()  [unwired: 2 in, 2 out]
                  }
                  frame 74 {
                    n409 = property on="Trigger histogram 74" class="XYGraph (strict)"("YScale.Maximum"=w455, "XScale.Minimum"=w454, "XScale.Maximum"=w453) -> ()  [unwired: 2 in, 2 out]
                  }
                  frame 75 {
                    n410 = property on="Trigger histogram 75" class="XYGraph (strict)"("YScale.Maximum"=w458, "XScale.Minimum"=w457, "XScale.Maximum"=w456) -> ()  [unwired: 2 in, 2 out]
                  }
                  frame 76 {
                    n411 = property on="Trigger histogram 76" class="XYGraph (strict)"("YScale.Maximum"=w461, "XScale.Minimum"=w460, "XScale.Maximum"=w459) -> ()  [unwired: 2 in, 2 out]
                  }
                  frame 77 {
                    n412 = property on="Trigger histogram 77" class="XYGraph (strict)"("YScale.Maximum"=w464, "XScale.Minimum"=w463, "XScale.Maximum"=w462) -> ()  [unwired: 2 in, 2 out]
                  }
                  frame 78 {
                    n413 = property on="Trigger histogram 78" class="XYGraph (strict)"("YScale.Maximum"=w467, "XScale.Minimum"=w466, "XScale.Maximum"=w465) -> ()  [unwired: 2 in, 2 out]
                  }
                  frame 79 {
                    n414 = property on="Trigger histogram 79" class="XYGraph (strict)"("YScale.Maximum"=w470, "XScale.Minimum"=w469, "XScale.Maximum"=w468) -> ()  [unwired: 2 in, 2 out]
                  }
                  frame 80 {
                    n415 = property on="Trigger histogram 80" class="XYGraph (strict)"("YScale.Maximum"=w473, "XScale.Minimum"=w472, "XScale.Maximum"=w471) -> ()  [unwired: 2 in, 2 out]
                  }
                  frame 81 {
                    n416 = property on="Trigger histogram 81" class="XYGraph (strict)"("YScale.Maximum"=w476, "XScale.Minimum"=w475, "XScale.Maximum"=w474) -> ()  [unwired: 2 in, 2 out]
                  }
                  frame 82 {
                    n417 = property on="Trigger histogram 82" class="XYGraph (strict)"("YScale.Maximum"=w479, "XScale.Minimum"=w478, "XScale.Maximum"=w477) -> ()  [unwired: 2 in, 2 out]
                  }
                  frame 83 {
                    n418 = property on="Trigger histogram 83" class="XYGraph (strict)"("YScale.Maximum"=w482, "XScale.Minimum"=w481, "XScale.Maximum"=w480) -> ()  [unwired: 2 in, 2 out]
                  }
                  frame 84 {
                    n419 = property on="Trigger histogram 84" class="XYGraph (strict)"("YScale.Maximum"=w485, "XScale.Minimum"=w484, "XScale.Maximum"=w483) -> ()  [unwired: 2 in, 2 out]
                  }
                  frame 85 {
                    n420 = property on="Trigger histogram 85" class="XYGraph (strict)"("YScale.Maximum"=w488, "XScale.Minimum"=w487, "XScale.Maximum"=w486) -> ()  [unwired: 2 in, 2 out]
                  }
                  frame 86 {
                    n421 = property on="Trigger histogram 86" class="XYGraph (strict)"("YScale.Maximum"=w491, "XScale.Minimum"=w490, "XScale.Maximum"=w489) -> ()  [unwired: 2 in, 2 out]
                  }
                  frame 87 {
                    n422 = property on="Trigger histogram 87" class="XYGraph (strict)"("YScale.Maximum"=w494, "XScale.Minimum"=w493, "XScale.Maximum"=w492) -> ()  [unwired: 2 in, 2 out]
                  }
                  frame 88 {
                    n423 = property on="Trigger histogram 88" class="XYGraph (strict)"("YScale.Maximum"=w497, "XScale.Minimum"=w496, "XScale.Maximum"=w495) -> ()  [unwired: 2 in, 2 out]
                  }
                  frame 89 {
                    n424 = property on="Trigger histogram 89" class="XYGraph (strict)"("YScale.Maximum"=w500, "XScale.Minimum"=w499, "XScale.Maximum"=w498) -> ()  [unwired: 2 in, 2 out]
                  }
                  frame 90 {
                    n425 = property on="Trigger histogram 90" class="XYGraph (strict)"("YScale.Maximum"=w503, "XScale.Minimum"=w502, "XScale.Maximum"=w501) -> ()  [unwired: 2 in, 2 out]
                  }
                  frame 91 {
                    n426 = property on="Trigger histogram 91" class="XYGraph (strict)"("YScale.Maximum"=w506, "XScale.Minimum"=w505, "XScale.Maximum"=w504) -> ()  [unwired: 2 in, 2 out]
                  }
                  frame 92 {
                    n427 = property on="Trigger histogram 92" class="XYGraph (strict)"("YScale.Maximum"=w509, "XScale.Minimum"=w508, "XScale.Maximum"=w507) -> ()  [unwired: 2 in, 2 out]
                  }
                  frame 93 {
                    n428 = property on="Trigger histogram 93" class="XYGraph (strict)"("YScale.Maximum"=w512, "XScale.Minimum"=w511, "XScale.Maximum"=w510) -> ()  [unwired: 2 in, 2 out]
                  }
                  frame 94 {
                    n429 = property on="Trigger histogram 94" class="XYGraph (strict)"("YScale.Maximum"=w515, "XScale.Minimum"=w514, "XScale.Maximum"=w513) -> ()  [unwired: 2 in, 2 out]
                  }
                  frame 95 {
                    n430 = property on="Trigger histogram 95" class="XYGraph (strict)"("YScale.Maximum"=w518, "XScale.Minimum"=w517, "XScale.Maximum"=w516) -> ()  [unwired: 2 in, 2 out]
                  }
                  frame 96 {
                    n431 = property on="Trigger histogram 96" class="XYGraph (strict)"("YScale.Maximum"=w521, "XScale.Minimum"=w520, "XScale.Maximum"=w519) -> ()  [unwired: 2 in, 2 out]
                  }
                  frame 97 {
                    n432 = property on="Trigger histogram 97" class="XYGraph (strict)"("YScale.Maximum"=w524, "XScale.Minimum"=w523, "XScale.Maximum"=w522) -> ()  [unwired: 2 in, 2 out]
                  }
                  frame 98 {
                    n433 = property on="Trigger histogram 98" class="XYGraph (strict)"("YScale.Maximum"=w527, "XScale.Minimum"=w526, "XScale.Maximum"=w525) -> ()  [unwired: 2 in, 2 out]
                  }
                  frame 99 {
                    n434 = property on="Trigger histogram 99" class="XYGraph (strict)"("YScale.Maximum"=w530, "XScale.Minimum"=w529, "XScale.Maximum"=w528) -> ()  [unwired: 2 in, 2 out]
                  }
                }
              }
            }
            event "Take image button": Mouse Down {
              w531 = FALSE
              n435 = event-data() -> ()  [unwired: 1 in, 7 out]
              n436 = flat-sequence {
                tunnel: [w533] -> w532
                tunnel: w532 -> [w543]
                frame #0 {
                  n437 = local read "ACQ full DATA file path"() -> (w539:path)
                  n438 = local read "Chip ID"() -> (w538:string)
                  n439 = Strip Path(path=w539) -> (stripped path=w536:path)  [unwired: 1 out]
                  n440 = Concatenate Strings(w538, "_ACQ_histograms.png" ("name or relative path")) -> (w534:string)
                  n441 = invoke class="VI" method="FP.Get Image"("image depth"=24 ("Image Depth")) -> ("image data"=w541:T3)  [unwired: 5 in, 5 out]
                  n442 = Build Path(base path=w536, name or relative path=w534) -> (appended path=w540:path)
                  n443 = call <vilib>:"Write PNG File.vi"("image data"=w541, "path to PNG file"=w540) -> ()  [unwired: 8 in, 2 out]
                  n444 = Concatenate Strings("Image saved\n", w534) -> (w533:string)
                }
                frame #1 {
                  n445 = call "MessageTimeOk.vi"("time (ms)"=2500, "missage"=w543) -> ()  [unwired: 4 in]
                }
              }
            }
          }
        }
      }
    }
  }
